vi "Window-Calibration toolbox_v9.vi"() -> ()   [LabVIEW 2020]
uses:
  Configuration code/Calibration/ToolBox/TypeDefs/Current Calibration Parameters.ctl
  Configuration code/Calibration/ToolBox/TypeDefs/ProcedureState.ctl
  Typedefs/Objective selector control enum.ctl
  <vilib>/vision/Image Controls.llb/IMAQ Image.ctl
  Configuration code/Calibration/ToolBox/TypeDefs/Incre-decr button.ctl
  Configuration code/Calibration/ToolBox/TypeDefs/Procedure_State.ctl
  Configuration code/Calibration/ToolBox/TypeDefs/Control Plane.ctl
  <vilib>/vision/Management.llb/Cast Image 2 Method.ctl
  Typedefs/HW config states enum.ctl
  Configuration code/Calibration/ToolBox/TypeDefs/data and image buffer fgv actions.ctl
  Typedefs/Shutter Function Enum.ctl
  Peripherals Control/XYZ Stage/Typedefs/XYZ stage data.ctl
  Peripherals Control/XYZ Stage/Typedefs/XYZ stage states.ctl
  Peripherals Control/XYZ Stage/Typedefs/XYZ channel ring.ctl
  Typedefs/Top level VI states.ctl
  Global Variables/General Globals.vi
  Configuration code/Calibration/Globals/gl_Calibration globals.vi
  Global Variables/gl_UI Ctrl Refs.vi
  <resource>/objmgr/IMAQImage.rc
  <vilib>/GPower/Array/GPArray.lvlib
  Global Variables/gl_Queues.vi
  <vilib>/vision/NI_Vision_Development_Module.lvlib
  <vilib>/GPower/Array/Library/Create/Random/CreateRandomI8.vi
panel:
  in  "Operation":T1(ring)
  in  "Exit":bool
  in  "Z Norm":bool
  in  "Signal Channel":enum16{"Red", "Green"}(ring)
  in  "Current Objective":T2="Olympus  20X"
  in  "Tab 2":T3(tab) caption="Calibration Tab"
  in  "Tab Control":T4(tab)
  in  "Freeze Core Image":bool
  out "Core Image":T5(plugin-control)
  in  "Core image":cluster{"Numeric":dbl, "Numeric":dbl}(slide)={"Numeric"=0.0, "Numeric"=1810.4210526315792} scale=0.0..4095.0
  in  "CH2":bool caption="CH"
  in  "Filter Type":T6(ring)
  out "Mean Value":sgl format="%.2f"
  in  "Mov. Avg":bool
  out "Histogram":T7(graph)
  out "Core Image frozen":T5(plugin-control)
  in  "Frozen core image intensity":cluster{"Numeric":dbl, "Numeric":dbl}(slide)={"Numeric"=0.0, "Numeric"=1810.4210526315792} scale=0.0..4095.0
  out "Core Image Filtered":T5(plugin-control)
  in  "Core image filtered":cluster{"Numeric":dbl, "Numeric":dbl}(slide)={"Numeric"=0.0, "Numeric"=1810.4210526315792} scale=0.0..255.0
  in  "AOL Controls Tab":T8(tab)
  in  "FOV":sgl(slide)=100.0 min=10 max=500 step=1 scale=25.0..500.0
  in  "Frame size":u16(slide)=256 min=2 max=2048 step=1 scale=2.0..2048.0
  in  "Dwell Time":dbl(slide)=0.1 min=0.05 max=0.4 step=0.05 scale=0.05..0.4
  in  "X Centre":sgl(slide) scale=-1.0..1.0 scale format="%#_2f"
  in  "Y Centre":sgl(slide) caption="Y centre" scale=-1.0..1.0 scale format="%#_2f"
  in  "AOLZ":sgl(slide) scale=-300.0..300.0 scale format="%#_2f"
  in  "Sum X":T9 step=0.1
  in  "Sum Y":T9 step=0.1
  in  "Sums Incr":dbl=0.1 caption="+/-" step=0.1
  in  "Diff X":T9 step=0.1
  in  "Diff Y":T9 step=0.1
  in  "Diffs Incr":dbl=0.1 caption="+/-"
  in  "Distortion Corr.":T9 step=0.1
  in  "DC Incr":dbl=0.1 caption="+/-"
  in  "X Angle":dbl(knob) min=0.0 max=359.9 step=0.1
  in  "Y Angle":dbl(knob)
  in  "Z Angle":dbl(knob)
  in  "Current Calibration Parameters":T10 {"Slip Cycle" step=0.1; "Samples to Wait after Trigger" step=0.1; "X_norm to um_scaling" step=0.1; "Z_norm to um_scaling" step=0.1; "Distortion Correction" step=0.1; "Diff Y" step=0.1; "Diff X" step=0.1; "Sum Y" step=0.1; "Sum X" step=0.1}
  in  "Incr":dbl=0.1 caption="+/-"
  in  "Plot":bool
  in  "Sort":bool
  in  "By":enum16{"Z", "X", "Y"}(ring)
  in  "Core Intensity 2":T11(tab) caption="Calibration Tab"
  out "Intensity":i16[][](graph)
  in  "Intensity Graph colour palette":cluster{dbl, "Color Box":u32}[](array[cluster])=[{1000.0, "Color Box"=16714752}, {750.0, "Color Box"=15859456}, {500.0, "Color Box"=65289}, {250.0, "Color Box"=983260}, {0.0, "Color Box"=14418124}]
  in  "core Intensity Graph colour palette":cluster{dbl, "Color Box":u32}[](array[cluster])=[{1000.0, "Color Box"=16714752}, {750.0, "Color Box"=15859456}, {500.0, "Color Box"=65289}, {250.0, "Color Box"=983260}, {0.0, "Color Box"=14418124}]
  out "Core Intensity":i16[][](graph)
  in  "Add images to buffer":bool
  in  "Saved Pos":i32[](listbox)
  in  "Add reference":bool
  in  "Clear all":bool
  in  "Clear selected":bool
  in  "Save to file":bool
  in  "Measure":bool
  in  "Tab Control 2":enum32{"Page 1", "Page 2"}(tab)
  out "Frozen image":T5(plugin-control)
  in  "Frozen Image intensity":cluster{i16, i16}(slide)={0, 2048} scale=0.0..4095.0
  in  "Image Buffer 1":i32(listbox)
  in  "Snap save":bool
  in  "Sweep":enum16{"Dwell Time", "SWAT"}(ring)
  out "Y Scaling":cluster{"X":dbl, "Y":dbl}[](graph)
  out "X Scaling":cluster{"X":dbl, "Y":dbl}[](graph)
  out "Z Scaling":cluster{"X":dbl, "Y":dbl}[](graph)
  in  "Reload":bool
  in  "Save config.ini":bool
  out "X":sgl format="X:%#_g"
  out "Y":sgl format="Y:%#_g"
  out "Z":sgl format="Z:%#_g"
  out "Procedure":T12
  out "Z plane exec time":u32
  out "error out 7":errorcluster
  out "error out 6":errorcluster
  out "Circles Data":T13(array[cluster])
  out "error out 8":errorcluster
  out "error out 5":errorcluster
  out "error out 3":errorcluster
  out "error out 4":errorcluster
  out "error out 2":errorcluster
  out "error out 10":errorcluster
  in  "Calibrate":bool
  in  "Test":bool
  in  "Sequence":bool
  in  "miniStep size":dbl=100.0 format="%#_g µm"
  out "UL":dbl=100.0 format="%#_g µm"
  out "LL":dbl=100.0 format="%#_g µm"
  out "mini steps":dbl=100.0
  out "New Image":T5
  in  "Freeze and plot":bool
  in  "sample dtype":dbl
  out "Stage Zeroed ?":bool
  out "Motor Z values":i32[](array[numeric])
  out "AOL Z values":i32[](array[numeric])
  out "Stage Zeroed ? 2":bool
  in  "Freeze Image":bool
  out "LB data full":string[][](array[string])
  out "LB data":string[][](array[string])
  out "Nb Circles":i32
  out "error out 9":errorcluster
  out "Intensity Graph":i16[][](graph)
  out "Image Pixels (I16)":i16[][](array[numeric])
  out "Progress":u8(slide) scale=0.0..21.0
  out "error out":errorcluster
  in  "Auto Focus":bool
  in  "Message_FrontPanel":string
  in  "Cancel":bool
  in  "Abort":bool
  in  "Next":bool
  in  "N":i32=512
  out "Stop_Ind":bool
  in  "Calibration Tab":T14(tab)
  in  "CH1":bool caption="CH"
  in  "Overlay\ncore":bool
  in  "Live Image intensity":cluster{i16, i16}(slide)={0, 2048} scale=0.0..4095.0
  in  "Visible(Grid)":bool
  in  "Grid Lines":u32=2 min=2 max=10 step=1
  out "Image":T5(plugin-control)
  out "Focal Plane":sgl format="Z:%#_g"
  in  "Set focal plane":bool
  in  "Natural Plane":bool
  in  "Move Up":bool
  in  "Move Down":bool
  in  "Z Step Size":dbl=100.0 format="%#_g µm"
  out "Stage XYZ Position":cluster{"X":sgl, "Y":sgl, "Z":sgl}
  in  "Zero Stage":bool
  out "X Res.":i32
  out "Y Res.":i32
  in  "Up":bool
  in  "Left":bool
  in  "Right":bool
  in  "Down":bool
  in  "Return":bool
  in  "XY Step Size":dbl=100.0 format="%#_g µm"
  in  "Core extraction size":i32 caption="Core size"
  in  "X offset":i32
  in  "Y offset":i32
  out "Array":T5[](array[plugin-control])
  out "Analysis Graph":cluster{"X":dbl, "Y":dbl}[](graph)
  out "PSF Plot":cluster{"X":dbl, "Y":dbl}[](graph)
  out "PSF Image":T5(plugin-control)
  in  "Objectives":string(tree)
  out "String":string
  out "Calibration.ini Path":path
  out "Calibration.ini":string
  in  "Step details":string
  in  "Step No":T15(ring)
  in  "Pockels Cell Value for pointing mode":dbl
  in  "auto-set pockel":bool
  in  "Calibration_min":dbl
  in  "Calibration_max":dbl
  in  "Search_min":dbl
  in  "Search_max":dbl
  in  "Testing Range (Norm)_max":dbl=1.0
  in  "Testing Range (Norm)_min":dbl=-1.0
  in  "Auto Calibration":bool
  in  "Measure PSF":bool
  in  "Calibration test type":T16(ring)
  in  "Calibration type":T17(ring)
  # "PROTOTYPE ONLY"
  # "This utility is under development, please report any \nissues to the contact details provided on github"
  # "12"
  # "0"
  # "2"
  # "8"
  # "0"
  # "2"
  # "PLACEHOLDER"
  # "Note :  Files will be saved in C:\\Support Files\\Calibration Data directory\nin pos_data_{date}_{time}.csv format"
  # "Current XYZ Stage Position"
  # "Natural Focal Plane Z motor position must\n be set to Zero before starting."
  # "Calibration Options"
  # "Maximal Search Range"
  # "to"
  # "(for sums &\ndiffs only)"
  # "Calibration Range from"
  # "to"
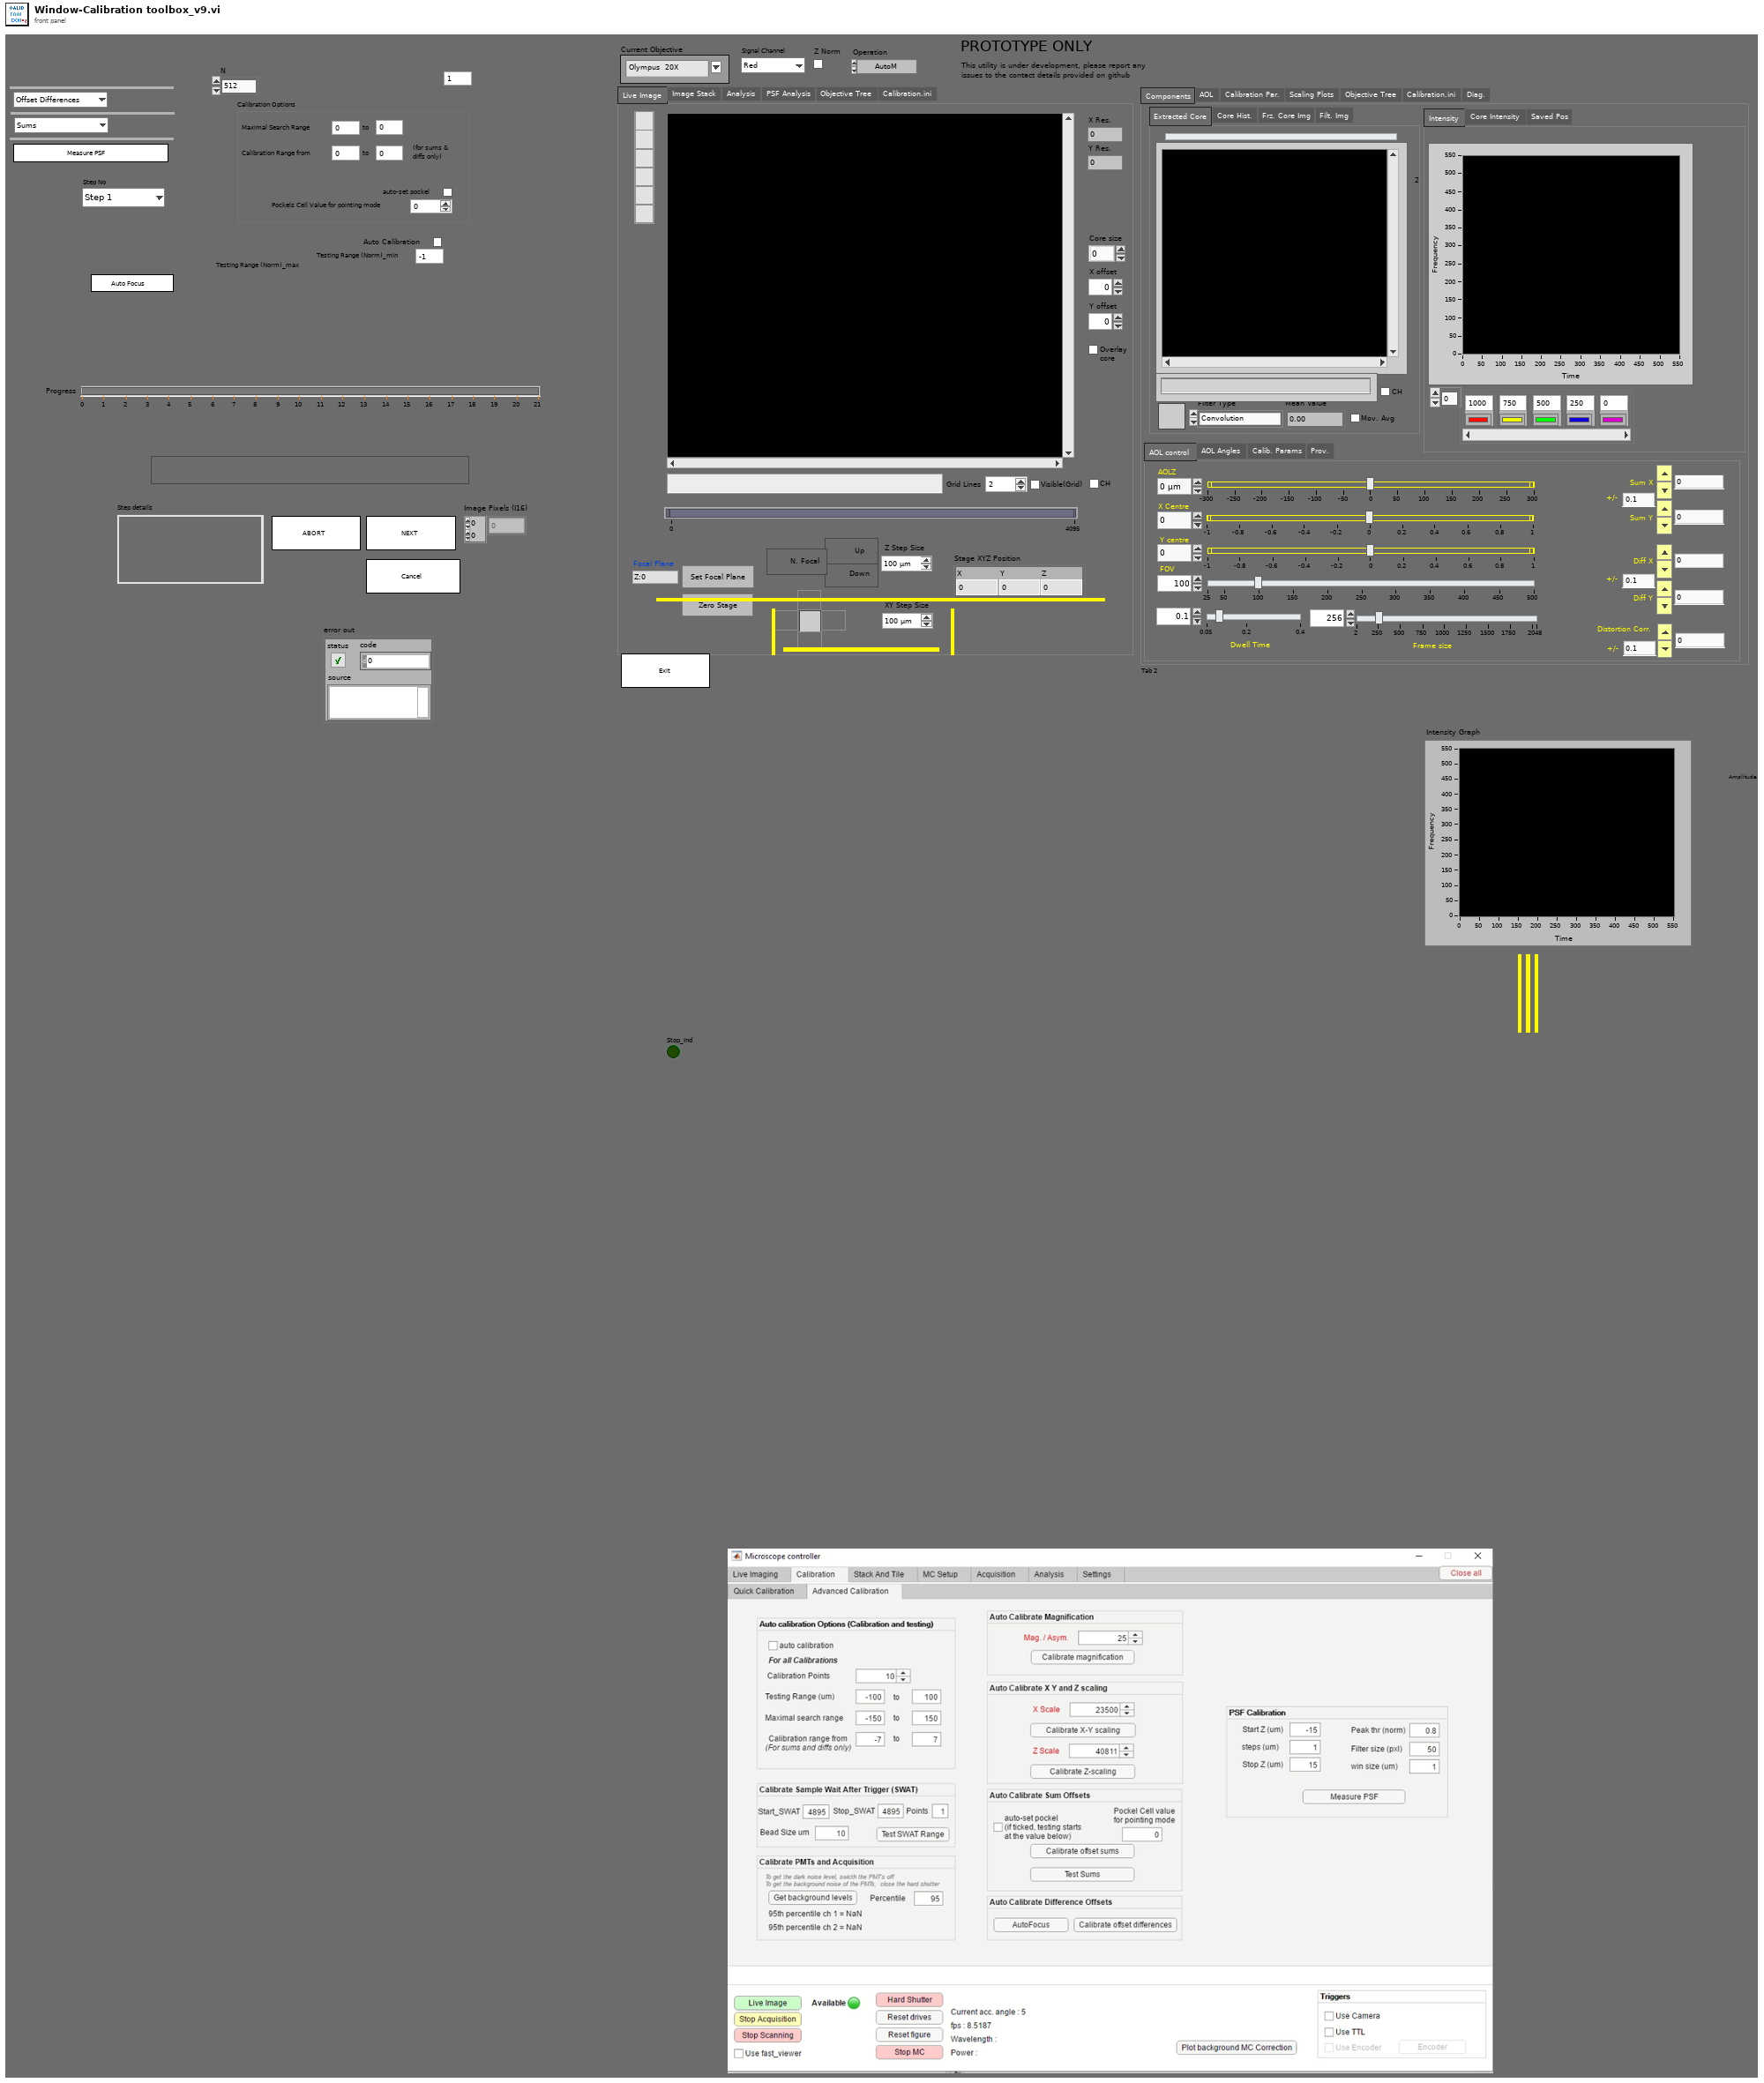
[diagram p1: front panel]
types:
  T1 = enum32{"AutoM", "Close", "Dilate", "Erode", "Gradient", "Gradient out", "Gradient in", "Hit miss", "Open", "PClose", "POpen", "Thick", "Thin"}
  T2 = typedef "Objective selector control enum.ctl" = string
  T3 = enum32{"Components", "AOL", "Calibration Par.", "Scaling Plots", "Objective Tree", "Calibration.ini", "Diag."}
  T4 = enum32{"Extracted Core", "Core Hist.", "Frz. Core Img", "Filt. Img"}
  T5 = typedef "IMAQ Image.ctl" = refnum<image>
  T6 = enum16{"Convolution", "Differentiation", "Gradient", "Prewitt", "Roberts", "Sigma", "Sobel"}
  T7 = cluster{"Starting Value":sgl, "Incremental Value":sgl, "Histogram":u32[]}
  T8 = enum32{"AOL control", "AOL Angles", "Calib. Params", "Prov."}
  T9 = typedef "Incre-decr button.ctl" = dbl
  T10 = typedef "Current Calibration Parameters.ctl" = cluster{"Sum X":dbl, "Sum Y":dbl, "Diff X":dbl, "Diff Y":dbl, "Distortion Correction":dbl, "Z_norm to um_scaling":dbl, "X_norm to um_scaling":dbl, "Samples to Wait after Trigger":dbl, "Slip Cycle":dbl}
  T11 = enum32{"Intensity", "Core Intensity ", "Saved Pos"}
  T12 = typedef "ProcedureState.ctl" = enum16{"Measure", "Calibrate", "Sequence", "Test"}
  T13 = cluster{"Pos. X":i32, "Pos. Y":i32, "Radius":i32, "Core Area":i32}[]
  T14 = enum32{"Live Image", "Image Stack", "Analysis", "PSF Analysis", "Objective Tree", "Calibration.ini"}
  T15 = enum16{"Step 1", "Step 2", "Step 3", "Step 4", "Step 5", "Step 6", "Step 7", "Step 8", "Step 9"}
  T16 = enum16{"Sums", "Diffs and Distortion", "Dwell Times"}
  T17 = enum16{"Offset Differences", "Magnification", "Offset Sums", "X-Y Scaling", "Z-Scaling"}
  T18 = typedef "Image Type" = u32
  T19 = enum32{"Invalid", "Standard", "Closed", "Hidden", "Minimized", "Maximized"}
  T20 = typedef "data and image buffer fgv actions.ctl" = enum16{"Initialise", "Add Image to buffer", "Read Image buffer", "Edit specific data", "Delete selected image", "Clear all images"}
  T21 = typedef "HW config states enum.ctl" = enum16{"Load from file", "Save to file", "Save backup", "Write all", "Read all", "Write XY stage settings", "Write DAQ FPGA settings", "Write Control FPGA settings", "Write Phys Channels", "Write System Config", "Write HW Config", "Save System Config", "Save HW Config", "Clear", "Compare from file"}
  T22 = enum8{"Enabled", "Disabled", "Disabled and Grayed Out"}
  T23 = enum16{"Initialise", "Load from file", "Save to file", "Read", "Write"}
  T24 = typedef "Shutter Function Enum.ctl" = enum16{"Open Shutter", "Close Shutter"}
  T25 = enum32{"Bad", "Idle", "Run top level", "Running"}
  T26 = typedef "Live graph data queue ref.ctl" = refnum<queue>
  T27 = enum32{"Image", "Image Stack", "Analysis", "PSF Analysis", "Objective Tree", "Calibration.ini"}
  T28 = typedef "Calibration config.ctl" = cluster{"Current Objective":string, "Objective Settings":T29[], "PreChirper Values Preset ?":bool, "PreChirper Settings":T30[], "PreChirper Constants":T31}
  T29 = typedef "Objective Config.ctl" = cluster{"Name":string, "Sum X":dbl, "Sum Y":dbl, "Diff X":dbl, "Diff Y":dbl, "Distortion Correction":dbl, "Z_norm to um_scaling":dbl, "X_norm to um_scaling":dbl, "Calibrated Wavelength":dbl}
  T30 = typedef "Prechirper Cal Config.ctl" = cluster{"Wavelength":i32, "Prism 1":i32, "Prism 2":i32}
  T31 = typedef "PreChirper constants.ctl" = cluster{"a 1":i32, "b 1":i32, "c 1":i32, "a 2":i32, "b 2":i32, "c 2":i32, "lmin":i32, "lmax":i32}
  T32 = typedef "System Configuration.ctl" = cluster{"Laser wavelength (nm)":dbl, "DAQ FPGA System":T33, "Control system":T34}
  T33 = typedef "DAQ FPGA system config.ctl" = cluster{"Clock Freq (MHz) ":dbl, "Samples Wait after Trigger":u16, "AOD fill":u16, "StartupDelay":i32, "Slip Cycle (clock cycles)":u32, "Add Cycle":bool}
  T34 = typedef "CTRL system config.ctl" = cluster{"AOD 1 Amplitude":i16, "AOD 2 Amplitude":i16, "AOD 3 Amplitude":i16, "AOD 4 Amplitude":i16, "AOD 5 Amplitude":i16, "AOD 6 Amplitude":i16, "T0 (ns)":dbl, "Ta (ns)":dbl, "Data Time Interval (ns)":dbl, "Ctrl FPGA Clock (MHz)":dbl}
  T35 = typedef "UI ctrl refs cluster.ctl" = cluster{"Top level VI path":path, "Top level VI ref":refnum<vi>, "User menu ref":refnum<k9>, "Sub Panel control":refnum<vi>, "Imaging Param Tab":refnum<vi>, "Occurrence-Start drivers":refnum<k4>, "Occurrence-Speed logging initialised":refnum<k4>, "Occurrence-XYZ stage initialised":refnum<k4>, "Exit button":refnum<vi>, "Status ind":refnum<vi>, "Set as origin":refnum<vi>, "Speed Logging":refnum<vi>, "Time Lapse":refnum<vi>, "Live Imaging":refnum<vi>, "AOL Z Stack":refnum<vi>, "Motor Z Stack":refnum<vi>, "Funct Acq button":refnum<vi>, "Hard Shutter":refnum<vi>, "Virtual Shutter":refnum<vi>, "Laser Power":refnum<vi>, "AOL Mode":refnum<vi>, "Frame Size":refnum<vi>, "Field of View":refnum<vi>, "Dwell Time":refnum<vi>, "Zoom":refnum<vi>, "AOL Z":refnum<vi>, "Objective":refnum<vi>, "Axis":refnum<vi>, "Paths & Names":refnum<vi>, "Experiment folder path (ind.)":refnum<vi>, "Last State (Ind.)":refnum<vi>, "Averages":refnum<vi>, "Angle (degrees)":refnum<vi>, "X centre":refnum<vi>, "Y centre":refnum<vi>, "Plane Mode":refnum<vi>, "# Planes":refnum<vi>, "Z Start":refnum<vi>, "Z Stop":refnum<vi>, "Z Step":refnum<vi>, "PMT 1":refnum<vi>, "PMT 2":refnum<vi>, "Stage XYZ Position":refnum<vi>, "Pockels@Z Start":refnum<vi>, "Pockels@Z Stop":refnum<vi>, "Obtain Z Start":refnum<vi>, "Obtain Z Stop":refnum<vi>, "Live stim.trig.period":refnum<vi>, "Live stim.trig.enable":refnum<vi>, "Movement Correction":refnum<vi>, "Load Reference Image":refnum<vi>, "XY Stage Move":refnum<vi>, "MovCor Cluster":refnum<vi>, "RefDAQParam":refnum<vi>, "Funct. Acq. Pockels Modulation":refnum<vi>, "Ref Laser Power":refnum<vi>, "Enable Video Recording":refnum<vi>, "Video Record-Live Imaging":refnum<vi>, "Video Record-Funct acq":refnum<vi>, "Reference Source":refnum<vi>, "AOL Z-stack Chirps Ready (ind)":refnum<vi>, "Target time between mov.cor. ref triggers (ms)":refnum<vi>, "Funct. Acq. Ref frame save":refnum<vi>, "Tracking button":refnum<vi>, "Show ref plots window":refnum<vi>, "Center freq ind (nm)":refnum<vi>, "Pickup mode (ind)":refnum<vi>, "Logging queue (ind)":refnum<vi>, "Back aperture power (ind.)":refnum<vi>, "Power after objective (ind.)":refnum<vi>, "Switch user":refnum<vi>, "Ls1 Conn. Status":refnum<vi>, "Ls1Tuning Status":refnum<vi>, "Ls1 Faults":refnum<vi>, "Ls1 Connection":refnum<vi>, "Ls1 Mode":refnum<vi>, "Ls1 POWER [mW]":refnum<vi>, "Ls1Shutter":refnum<vi>, "Ls1 Wavelength":refnum<vi>, "Ls1 Note":refnum<vi>, "Ls1 Confirm Wav":refnum<vi>, "Ls1 PreChrp Prism1":refnum<vi>, "Ls1 PreChrp Prism2":refnum<vi>, "Ls1 wav top Ind":refnum<vi>, "Ls1 power top Ind":refnum<vi>, "Ls1 Pump peak Hold":refnum<vi>, "Ls1 Status Ind":refnum<vi>, "Ls1 wav cancel":refnum<vi>, "Experiment Type":refnum<vi>, "Biology Information":refnum<vi>, "Camera recording status":refnum<vi>, "Optimise Obj. Pos.":refnum<vi>}
  T36 = typedef "AOL Z cal process refs.ctl" = cluster{"This VI":refnum<vi>, "Abort (ind)":refnum<vi>, "Next (ind)":refnum<vi>, "Cancel":refnum<vi>, "Next":refnum<vi>, "Message":refnum<vi>, "Progress":refnum<vi>}
  T37 = typedef "Frame Size.ctl" = u16
  T38 = typedef "Control Plane.ctl" = enum16{"XY-X", "XY-Y", "Z"}
  T39 = typedef "Procedure_State.ctl" = cluster{"Procedure":T12, "Parameter":T38, "Symmetric":bool}
  T40 = typedef "XYZ stage states.ctl" = enum16{"Dequeue", "Initialize", "Read Position", "Read Speed Setting", "Move", "Set Max Speed", "Reset Axis", "Stop all movement"}
  T41 = typedef "XYZ channel ring.ctl" = string
  T42 = typedef "XYZ stage data.ctl" = cluster{"Command":T40, "Channel":T41, "X":sgl, "Y":sgl, "Z":sgl, "Speed":i32, "Zero":bool, "Use acknowledgement?":bool}
  T43 = typedef "Top level VI states.ctl" = enum16{"None", "Initialise UI", "<STACK PROTOCOL STATES>", "AOL Zstack-START", "AOL Zstack-STOP", "Motor Zstack-START", "Motor Zstack-STOP", "Parameter Sweep-START", "Parameter Sweep-STOP", "<ACQUISITION PROTOCOL STATES> ", "Functional Acquisition-START", "Functional Acquisition-STOP", "Single Plane Acquisition-START", "Single Plane Acquisition-STOP", "Volume Acquisition-START", "Volume Acquisition-STOP", "<LIVE IMAGING PROTOCOL STATES>", "Live Imaging-START", "Live Imaging-STOP", "Live Plane Imaging-START", "Live Plane Imaging-STOP", "Live Volume Imaging-START", "Live Volume Imaging-STOP", "<MOVEMENT CORRECTION PROTOCOL STATES>", "EXIT"}
  T44 = enum16{"open", "replace", "create", "open or create", "replace or create", "replace or create with confirmation"}
  T45 = typedef "AOL_Globals.ctl" = cluster{"Imaging Protocol":T46, "Number of POI":u16, "Number of Miniscans":u16, "Number of Trials":u16, "Number of Cycles ":u64, "# Averaged Frames":u16, "Laser power (%)":u8, "Pockels (V)":dbl, "Acquisition Length (sec)":dbl, "Fill time (us)":dbl, "POI Dwell time (us)":dbl, "Miniscan Dwell time per pixel (us)":dbl, "PMT 1":dbl, "PMT 2":dbl, "Back Apperture (mA)":dbl, "Frame Size":T37, "Center Frequency":dbl, "Field of View (um)":dbl, "Field of View (norm)":dbl, "DwellTime (us)":dbl, "Ref Dwell Time (us)":dbl, "Wavelength (nm)":dbl, "Zoom":dbl, "AOL Z":dbl, "AOL Mode":T47, "GridXY":dbl, "GridZ":dbl, "TriggerPeriod (sec)":dbl, "Number of Pixels in Miniscan":u16, "Experiment folder path":path, "X centre":dbl, "Y centre":dbl, "Angle (degrees)":dbl, "Angle Xs (degrees)":dbl, "Angle Ys (degrees)":dbl, "Plane Mode":T48, "Threshold":u16[], "Regenerate Chirps":bool, "Rectangle ROI length (pixels)":u16, "Rectangle ROI height (pixels)":u16, "AOD fill":u16, "StartupDelay":i32, "Samples Wait after Trigger":u16, "Slip Cycle":u32, "Add Cycle":bool, "Functional Mode":T49, "Z Start":dbl, "Z Stop":dbl, "# Planes":i32, "Total Pixels":i32, "Variable Miniscan Pixels":u16[], "Use Variable Length":bool, "Use Variable Resolution":bool, "Laser power (%) at Z Start":u8, "Laser power (%) at Z Stop":u8, "Ref Z Step":i8}
  T46 = typedef "Imaging Protocols enum.ctl" = enum16{"AOL Z-Stack", "Motor Z Stack", "Parameter Sweep", "Functional Acquisition", "Single Plane Acquisition", "Volume Acquisition", "Live Imaging", "Live Plane Imaging", "Live Volume Imaging"}
  T47 = typedef "AOL modes.ctl" = enum16{"Raster", "Structural", "Pointing", "Mini Scan", "Alignment"}
  T48 = typedef "Plane Mode.ctl" = u16
  T49 = typedef "Functional Mode.ctl" = enum16{"Point", "Line", "Patch", "Plane", "Volume"}
  T50 = typedef "Live imaging queue element.ctl" = cluster{"Red channel":T5, "Green channel":T5, "Ref Red channel":T5, "Ref Green channel":T5, "Mov cor":bool}
  T51 = typedef "IMAQ Circle" = cluster{"Center X":i32, "Center Y":i32, "Inner Radius":i32, "Outer Radius":i32, "Start Angle":dbl, "End Angle":dbl}
  T52 = enum32{"Differentiation", "Gradient", "Prewitt", "Roberts", "Sigma", "Sobel"}
  T53 = typedef "Cast Image 2 Method.ctl" = u32
  T54 = typedef "ROI Descriptor" = cluster{"Global Rectangle":i32[], "Contours":cluster{"ID":enum32{"External", "Internal"}, "Type":u32, "Coordinates":i32[]}[]}
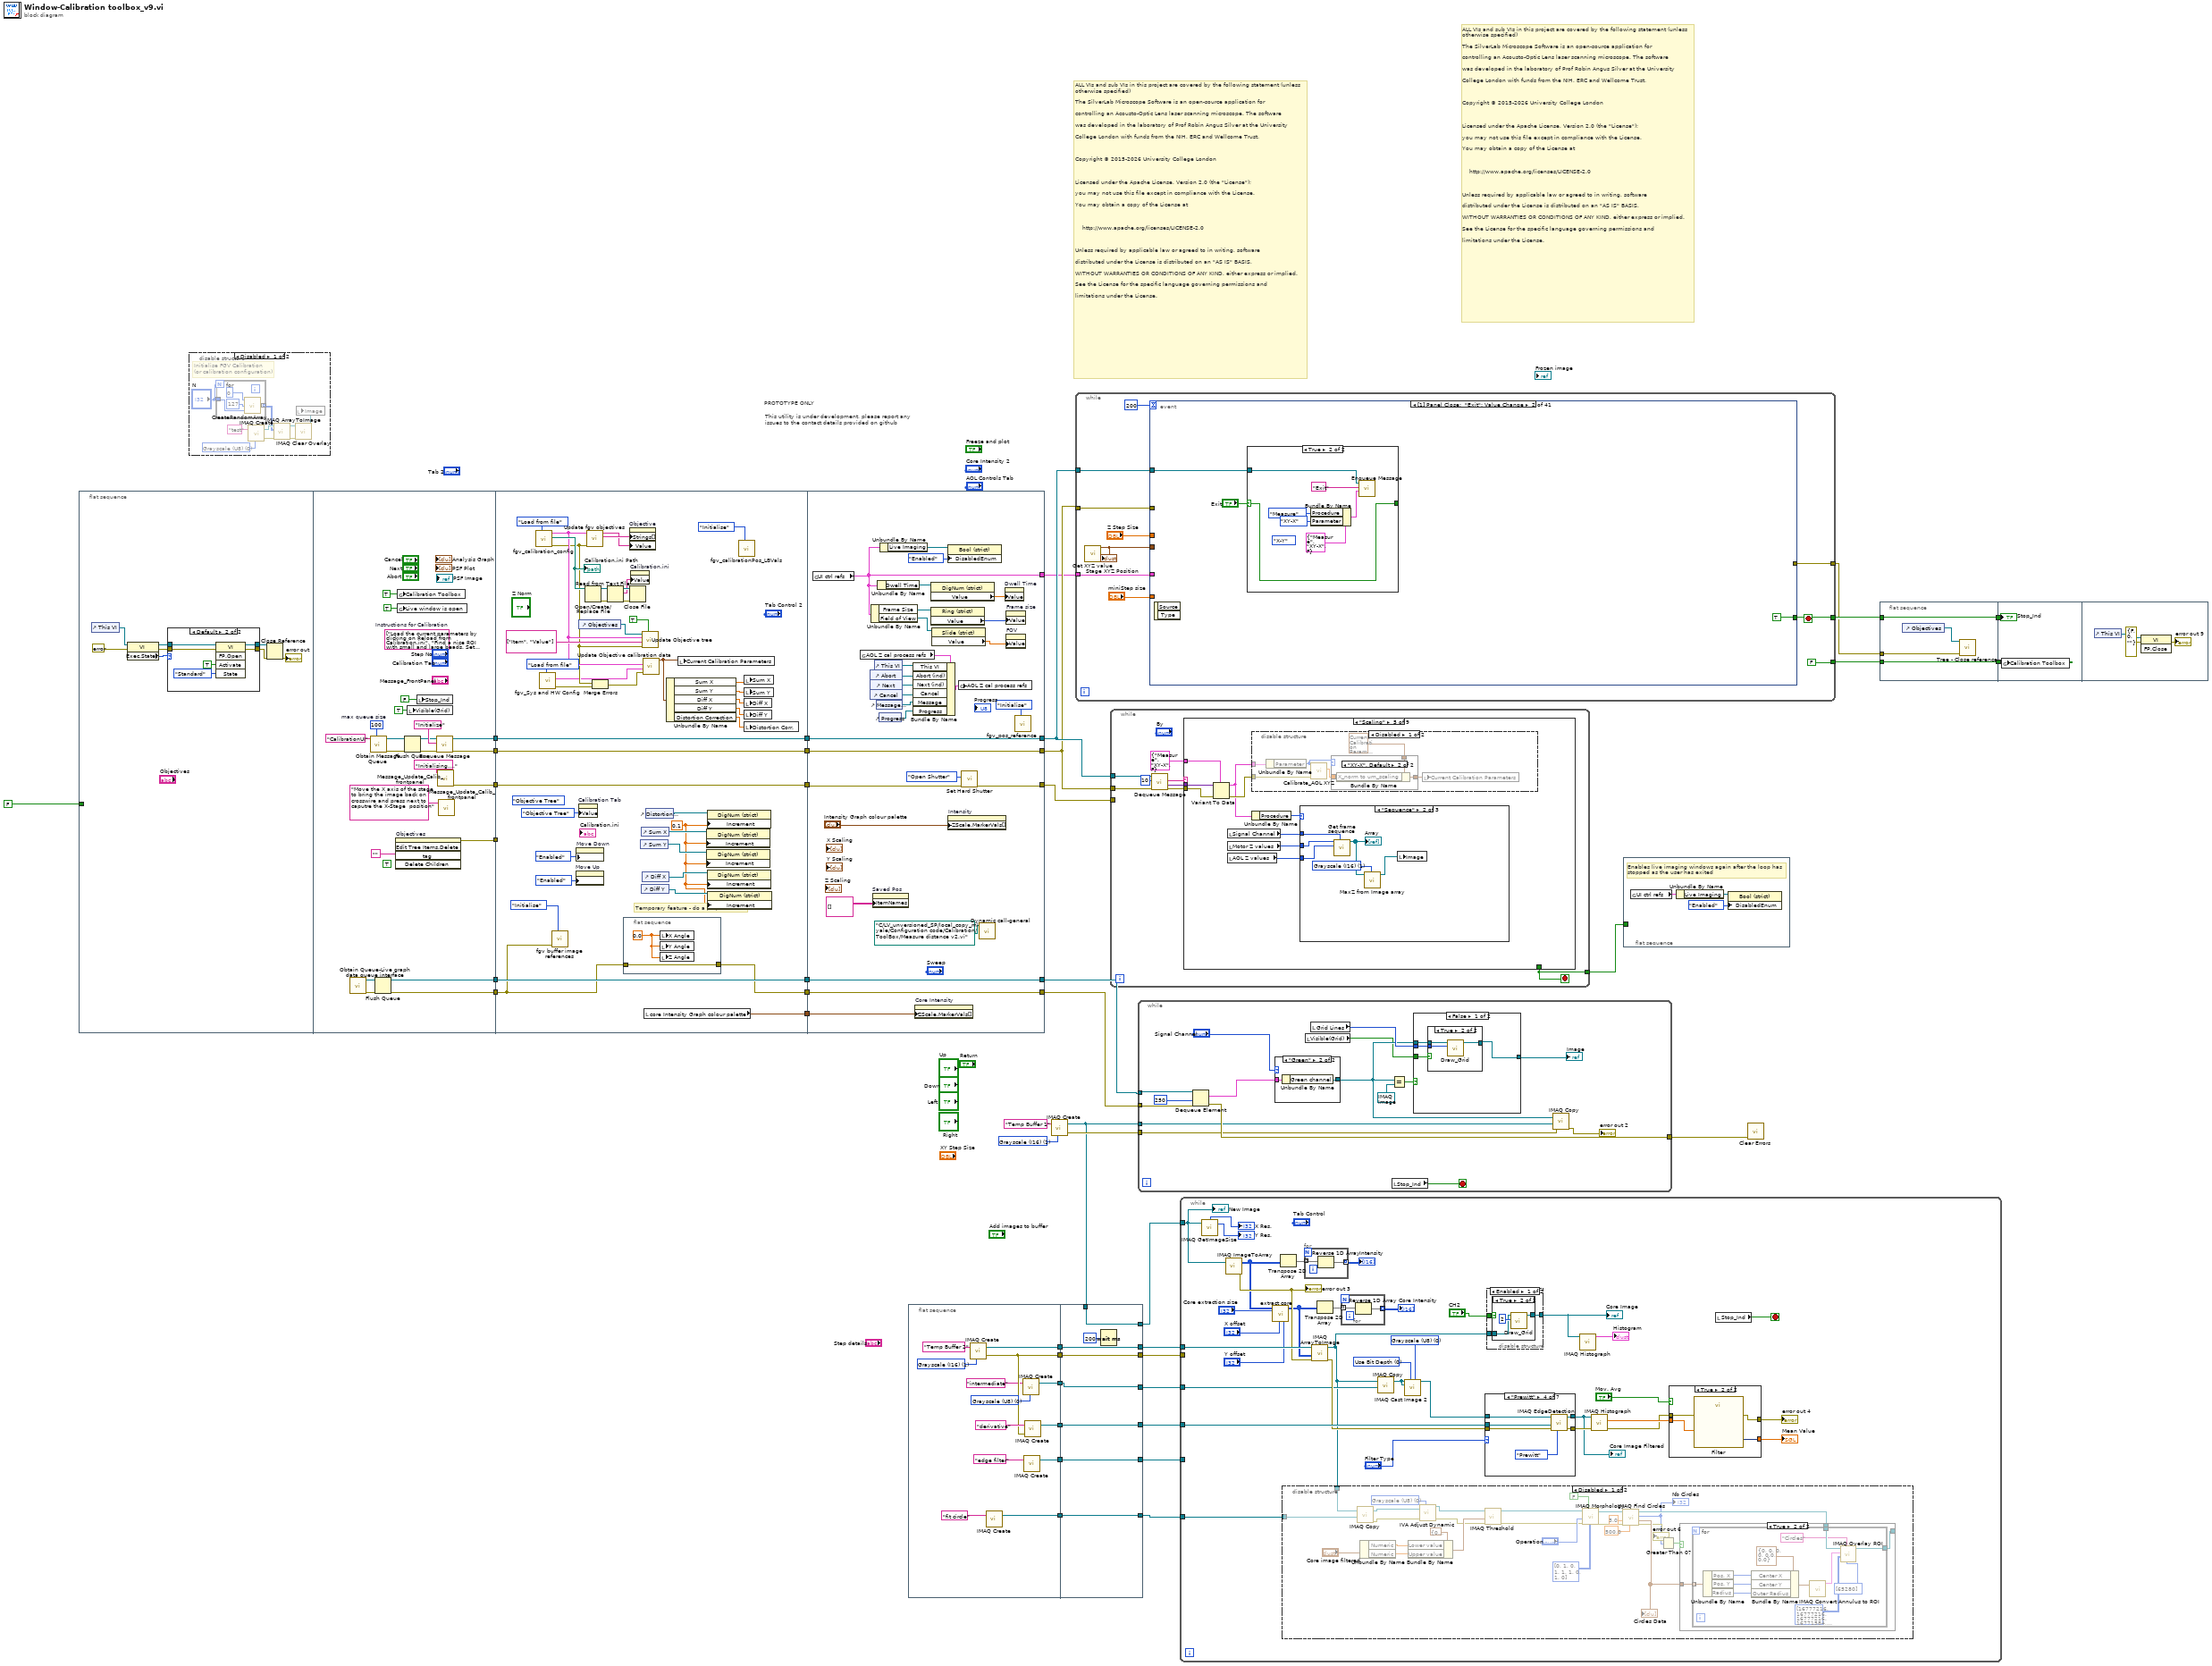
[diagram p0: block diagram]
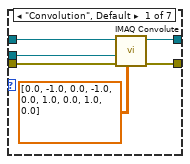
[diagram p7: hidden frame]
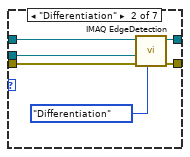
[diagram p8: hidden frame]
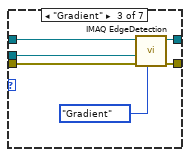
[diagram p9: hidden frame]
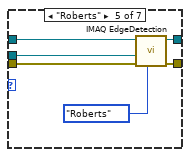
[diagram p10: hidden frame]
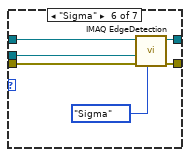
[diagram p11: hidden frame]
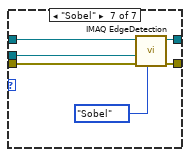
[diagram p12: hidden frame]
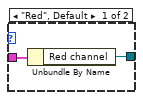
[diagram p14: hidden frame]
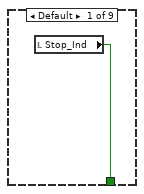
[diagram p18: hidden frame]
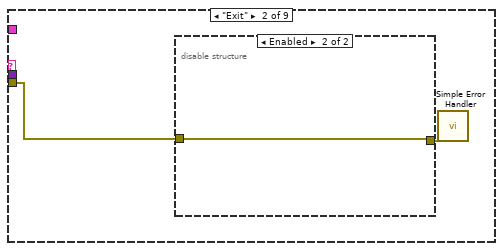
[diagram p19: hidden frame]
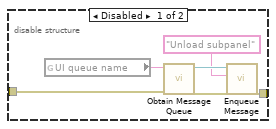
[diagram p20: hidden frame]
diagram:
  w23 = T18 1 items=["Grayscale (U8)", "Grayscale (I16)", "Grayscale (SGL)", "Complex (CSG)", "RGB (U32)", "HSL (U32)", "RGB (U64)", "Grayscale (U16)"] ("Image Type")
  # "ALL VIs and sub VIs in this project are covered by the following statement (unless \notherwise specified)\n\nThe SilverLab Microscope Software is an open-source application for\n\ncontrolling an Acousto-Optic Lens laser scanning microscope. The software\n\nwas developed in the laboratory of Prof Robin Angus Silver at the University\n\nCollege London with funds from the NIH, ERC and Wellcome Trust.\n\n \n\nCopyright © 2015-2026 University College London\n\n \n\nLicensed under the Apache License, Version 2.0 (the \"License\");\n\nyou may not use this file except in compliance with the License.\n\nYou may obtain a copy of the License at\n\n \n\n    http://www.apache.org/licenses/LICENSE-2.0\n\n \n\nUnless required by applicable law or agreed to in writing, software\n\ndistributed under the License is distributed on an \"AS IS\" BASIS,\n\nWITHOUT WARRANTIES OR CONDITIONS OF ANY KIND, either express or implied.\n\nSee the License for the specific language governing permissions and\n\nlimitations under the License."
  # "This utility is under development, please report any \nissues to the contact details provided on github"
  # "PROTOTYPE ONLY"
  # "ALL VIs and sub VIs in this project are covered by the following statement (unless \notherwise specified)\n\nThe SilverLab Microscope Software is an open-source application for\n\ncontrolling an Acousto-Optic Lens laser scanning microscope. The software\n\nwas developed in the laboratory of Prof Robin Angus Silver at the University\n\nCollege London with funds from the NIH, ERC and Wellcome Trust.\n\n \n\nCopyright © 2015-2026 University College London\n\n \n\nLicensed under the Apache License, Version 2.0 (the \"License\");\n\nyou may not use this file except in compliance with the License.\n\nYou may obtain a copy of the License at\n\n \n\n    http://www.apache.org/licenses/LICENSE-2.0\n\n \n\nUnless required by applicable law or agreed to in writing, software\n\ndistributed under the License is distributed on an \"AS IS\" BASIS,\n\nWITHOUT WARRANTIES OR CONDITIONS OF ANY KIND, either express or implied.\n\nSee the License for the specific language governing permissions and\n\nlimitations under the License."
  n1 = flat-sequence {
    tunnel: FALSE -> [_]
    tunnel: [w74] -> w37
    tunnel: [w73] -> w35
    tunnel: [w71] -> w33
    tunnel: [w64] -> w31
    tunnel: [w62] -> w29
    tunnel: [w61] -> w25
    tunnel: w37 -> [w123]
    tunnel: [w123] -> w36
    tunnel: w35 -> [w122]
    tunnel: [w122] -> w34
    tunnel: w33 -> [w121]
    tunnel: [w121] -> w32
    tunnel: w31 -> [w120]
    tunnel: [w120] -> w30
    tunnel: w29 -> [w84]
    tunnel: [w91] -> w28
    tunnel: w25 -> [_]
    tunnel: [w98] -> w19
    tunnel: [w151] -> w17
    tunnel: [w152] -> w18
    tunnel: [w132] -> w39
    tunnel: [w153] -> w41
    tunnel: [w154] -> w42
    tunnel: w36 -> [w154]
    tunnel: w34 -> [w153]
    tunnel: w32 -> [w133]
    tunnel: w30 -> [w152]
    tunnel: w28 -> [w151]
    tunnel: [w131] -> w27
    tunnel: w19 -> [w139]
    frame #0 {
      n2 = control-ref of="This VI"() -> (w48:refnum<vi>)
      n3 = property class="VI"(reference=w48, error in=errorcluster {"status"=FALSE, "code"=0, "source"=""} ("error in (no error)")) -> (reference out=w47:refnum<vi>, error out=w46:errorcluster, "Exec.State"=w44:T25)
      n4 = case shown="Default" w44 {
        tunnel: [w53 w54] -> w51
        tunnel: [w52 w59] -> w50
        tunnel: w47 -> [w53 w56]
        tunnel: w46 -> [w52 w55]
        frame "Run top level" {
        }
        frame Default {
          n5 = invoke class="VI" method="FP.Open"(reference=w56, error in=w55, "Activate"=TRUE ("Activate?"), "State"=T19."Standard") -> (reference out=w54:refnum<vi>, error out=w59:errorcluster)  [unwired: 1 in, 3 out]
        }
      }
      n6 = Close Reference(reference=w51, error in (no error)=w50) -> (error out=→"error out":errorcluster)
    }
    frame #1 {
      (unwired) TRUE ("Delete Children?")
      w76 = 100  # max queue size
      (unwired) string[] ["Load the current parameters by clicking on Reload from Calibration.ini", "Find a nice ROI with small and large beads. Set PMT at 500 and adjust pockels", "Test FOV gives a sharp, single peak with Auto Focus. If yes, zero the stage. Otherwise change ROI", "Use 'Test Diffs and distortion' AND ' Test Sum' to see if the rig needs calibration for differences or sums.", "Process to teh necessary calibrations. If the performances are suboptimal, change ROI or incease laser", "If the results are bad, you can restore the previous settings by clicking on Reload from calibration.ini", "If calibration fails repetitively, try another magnification, laser pwer or FOV size.", "If calibration crashes in mid-process, go to Acquisition tab, reset drives and set the stage back to [0,0,0]. If you were in pointing mode, set teh mode toggie back to raster. Then check the pockels values."]  # Instructions for Calibration
      n7 = call "Obtain Queue-Live graph data queue interface.vi"() -> ("error out"=w65:errorcluster, "Live graphs queue"=w66:T26)  [unwired: 10 in]
      n8 = call "Obtain Message Queue.vi"("max queue size (-1, unlimited)"=w76, "Queue name"="CalibrationUI") -> ("error out"=w78:errorcluster, "Message Queue"=w80:refnum<queue>)  [unwired: 8 in]
      n9 = Flush Queue(queue=w66, error in (no error)=w65) -> (queue out=w64:T26, error out=w62:errorcluster)  [unwired: 1 out]
      n10 = invoke on="Objectives" class="Tree (strict)" method="Edit Tree Items.Delete"("tag"="") -> (error out=w61:errorcluster)  [unwired: 4 in, 4 out]
      n11 = global write "General Globals.vi" "Calibration Toolbox"(TRUE ("Calibration Toolbox")) -> ()
      n12 = global write "General Globals.vi" "Live window is open"(TRUE ("Live window is open")) -> ()
      n13 = Flush Queue(queue=w80, error in (no error)=w78) -> (queue out=w79:refnum<queue>, error out=w77:errorcluster)  [unwired: 1 out]
      n14 = local write "Visible(Grid)"(TRUE ("Visible(Grid)")) -> ()
      n15 = local write "Stop_Ind"(FALSE ("Stop_Ind")) -> ()
      n16 = call "Enqueue Message.vi"("error in (no error)"=w77, "Message"="Initialize", "Queue"=w79) -> ("error out"=w73:errorcluster, "Queue out"=w74:refnum<queue>)  [unwired: 7 in]
      n17 = call "Message_Update_Calib_frontpanel.vi"("Message"="Initialising....") -> ("error out"=w71:errorcluster)  [unwired: 10 in]
      n18 = call "Message_Update_Calib_frontpanel.vi"("Message"="Move the X axis of the stage to bring the image back on crosswire and press next to caputre the X-Stage  position") -> ()  [unwired: 10 in, 1 out]
    }
    frame #2 {
      w85 = 0.1 ("Data Entry Limits:Increment")
      (unwired) T27."Objective Tree" ("Calibration Tab")
      # "Temporary feature - do a proper initialise"
      n19 = call "fgv_calibration_config.vi"("Cal config ops"=T23."Load from file") -> ("error out"=w103:errorcluster, "Config file path"=w108:path, "Config cluster OUT"=w107:T28)  [unwired: 8 in]
      "Calibration.ini Path" <- w108
      n20 = call "fgv_Sys and HW Config.vi"("Function"=HW_config_states_enum."Load from file") -> ("error out"=w102:errorcluster, "System Config OUT"=w100:T32)  [unwired: 8 in, 1 out]
      n21 = call "fgv buffer image references.vi"("Actions"=data_and_image_buffer_fgv_actions."Initialise", "error in (no error)"=w84) -> ()  [unwired: 7 in, 7 out]
      n22 = property on="Move Up" class="Bool"("DisabledEnum"=T22."Enabled" ("Disabled")) -> ()  [unwired: 2 in, 2 out]
      n23 = property on="Move Down" class="Bool"("DisabledEnum"=T22."Enabled" ("Disabled")) -> ()  [unwired: 2 in, 2 out]
      n24 = property on="Calibration Tab" class="TabCtl (strict)"("Value"=T14."Objective Tree" ("Calibration Tab")) -> ()  [unwired: 2 in, 2 out]
      n25 = control-ref of="Objectives"() -> (w111:refnum<vi>)
      n26 = Open/Create/Replace File(file path (use dialog)=w108) -> (refnum out=w116:refnum<file>, error out=w115:errorcluster)  [unwired: 5 in, 1 out]
      n27 = call "Update fgv objectives.vi"("error in (no error)"=w103, "Config cluster IN"=w107) -> ("Available Objectives"=w113:string[], "Current Objective"=w112:string)  [unwired: 7 in, 1 out]
      n28 = Merge Errors(w103, w102) -> (w101:errorcluster)
      n29 = Read from Text File(file (use dialog)=w116, error in=w115) -> (refnum out=w117:refnum<file>, text=w114:string, error out=w118:errorcluster)  [unwired: 2 in, 1 out]
      n30 = flat-sequence {
        tunnel: [w124] -> w91
        tunnel: w84 -> [w124]
        frame #0 {
          w125 = 0.0
          n31 = local write "X Angle"(w125) -> ()
          n32 = local write "Y Angle"(w125) -> ()
          n33 = local write "Z Angle"(w125) -> ()
        }
      }
      n34 = property on="Objective" class="CmbBox (strict)"("Strings[]"=w113, "Value"=w112) -> ()  [unwired: 2 in, 2 out]
      n35 = Close File(refnum=w117, error in=w118) -> ()  [unwired: 2 out]
      n36 = property on="Calibration.ini" class="Str"("Value"=w114) -> ()  [unwired: 2 in, 2 out]
      n37 = control-ref of="Sum Y"() -> (w86:refnum<vi>)
      n38 = control-ref of="Sum X"() -> (w87:refnum<vi>)
      n39 = control-ref of="Diff Y"() -> (w88:refnum<vi>)
      n40 = call "Update Objective tree.vi"("Visible Items:Column Headers Visible"=TRUE, "error in (no error)"=w103, "Column Header Strings[]"=string[] ["Item", "Value"], "Config cluster IN"=w107, "TreeControl in"=w111) -> ()  [unwired: 6 in, 1 out]
      n41 = control-ref of="Diff X"() -> (w89:refnum<vi>)
      n42 = call "Update Objective calibration data.vi"("error in (no error)"=w101, "System Config"=w100, "Config cluster OUT"=w107) -> ("Current Calibration Parameters out"=w97:T10)  [unwired: 7 in, 1 out]
      n43 = local read "core Intensity Graph colour palette"() -> (w98:cluster{dbl, "Color Box":u32}[])
      n44 = control-ref of="Distortion Corr."() -> (w90:refnum<vi>)
      n45 = Unbundle By Name(w97) -> ("Sum X"=w96:dbl, "Sum Y"=w95:dbl, "Diff X"=w94:dbl, "Diff Y"=w93:dbl, "Distortion Correction"=w92:dbl)
      n46 = local write "Current Calibration Parameters"(w97) -> ()
      n47 = property class="DigNum (strict)"(reference=w87, "Increment"=w85) -> ()  [unwired: 1 in, 2 out]
      n48 = property class="DigNum (strict)"(reference=w86, "Increment"=w85) -> ()  [unwired: 1 in, 2 out]
      n49 = property class="DigNum (strict)"(reference=w90, "Increment"=w85) -> ()  [unwired: 1 in, 2 out]
      n50 = property class="DigNum (strict)"(reference=w89, "Increment"=w85) -> ()  [unwired: 1 in, 2 out]
      n51 = property class="DigNum (strict)"(reference=w88, "Increment"=w85) -> ()  [unwired: 1 in, 2 out]
      n52 = call "fgv_calibrationPos_LBVals.vi"("ACtions"=enum16{"Initialise", "Get", "Set"}."Initialise") -> ()  [unwired: 9 in, 2 out]
      n53 = local write "Sum X"(w96) -> ()
      n54 = local write "Sum Y"(w95) -> ()
      n55 = local write "Diff X"(w94) -> ()
      n56 = local write "Diff Y"(w93) -> ()
      n57 = local write "Distortion Corr."(w92) -> ()
    }
    frame #3 {
      n58 = global read "gl_UI Ctrl Refs.vi" "UI ctrl refs"() -> (w131:T35)
      n59 = global read "gl_Calibration globals.vi" "AOL Z cal process refs"() -> (w145:T36)
      n60 = control-ref of="Abort"() -> (w144:refnum<vi>)
      n61 = control-ref of="Next"() -> (w150:refnum<vi>)
      n62 = control-ref of="Cancel"() -> (w146:refnum<vi>)
      n63 = Unbundle By Name(w131) -> ("Frame Size"=w130:refnum<vi>, "Field of View"=w128:refnum<vi>)
      n64 = property on="Saved Pos" class="MCListbox (strict)"("ItemNames"=string[][] []) -> ()  [unwired: 2 in, 2 out]
      n65 = control-ref of="This VI"() -> (w149:refnum<vi>)
      n66 = control-ref of="Message_FrontPanel"() -> (w147:refnum<vi>)
      n67 = Unbundle By Name(w131) -> ("Dwell Time"=w136:refnum<vi>)
      n68 = control-ref of="Progress"() -> (w141:refnum<vi>)
      n69 = Unbundle By Name(w131) -> ("Live Imaging"=w143:refnum<vi>)
      n70 = Bundle By Name(cluster=w145, "This VI"=w149, "Abort (ind)"=w144, "Next (ind)"=w150, "Cancel"=w146, "Message"=w147, "Progress"=w141) -> (w148:T36)
      n71 = property on="Core Intensity" class="IntGraph (strict)"("ZScale.MarkerVals[]"=w139) -> ()  [unwired: 2 in, 2 out]
      n72 = property class="DigNum (strict)"(reference=w136) -> ("Value"=w135:dbl)  [unwired: 1 in, 2 out]
      n73 = property class="Ring (strict)"(reference=w130) -> ("Value"=w129:T37)  [unwired: 1 in, 2 out]
      n74 = property class="Slide (strict)"(reference=w128) -> ("Value"=w127:sgl)  [unwired: 1 in, 2 out]
      n75 = property class="Bool (strict)"(reference=w143, "DisabledEnum"=T22."Enabled" ("Disabled")) -> ()  [unwired: 1 in, 2 out]
      n76 = property on="Intensity" class="IntGraph (strict)"("ZScale.MarkerVals[]"="Intensity Graph colour palette") -> ()  [unwired: 2 in, 2 out]
      n77 = global write "gl_Calibration globals.vi" "AOL Z cal process refs"(w148) -> ()
      n78 = call "Set Hard Shutter.vi"("Error In"=w133, "Shutter Function"=Shutter_Function_Enum."Open Shutter") -> ("Error Out"=w132:errorcluster)  [unwired: 9 in]
      n79 = call "Dynamic call-general.vi"("vi path"=path "C:/LV_unversioned_SP/local_copy_ml_yale/Configuration code/Calibration/ToolBox/Measure distance v2.vi") -> ()  [unwired: 10 in, 1 out]
      n80 = property on="Dwell Time" class="Slide (strict)"("Value"=w135) -> ()  [unwired: 2 in, 2 out]
      n81 = property on="Frame size" class="Slide (strict)"("Value"=w129) -> ()  [unwired: 2 in, 2 out]
      n82 = property on="FOV" class="Slide (strict)"("Value"=w127) -> ()  [unwired: 2 in, 2 out]
      n83 = call "fgv_pos_reference.vi"("State"=enum16{"Initialise", "Write", "Read", "Clear"}."Initialise") -> ()  [unwired: 8 in, 3 out]
    }
  }
  n84 = disable-structure shown="Disabled" {
    frame Disabled {
      w162 = T18 0 items=["Grayscale (U8)", "Grayscale (I16)", "Grayscale (SGL)", "Complex (CSG)", "RGB (U32)", "HSL (U32)", "RGB (U64)", "Grayscale (U16)"] ("Image Type")
      # "Initialise FGV Calibration\n(or calibration configuration)"
      n85 = for {
        N: "N" -> [_]
        tunnel: [w165] -> w159 mode=indexing
        tunnel: "N" -> [w164]
        n86 = call-poly <vilib>:"CreateRandomArray.vi"("N"=w164, "Maximum value"=i8 127, "Minimum value"=i8 0) -> ("Created array"=w165:i8[])
      }
      n87 = call "IMAQ Create"("Image Name"="test", "Image Type"=w162) -> ("New Image"=w160:T5, "error out"=w161:errorcluster)  [unwired: 3 in]
      n88 = call "IMAQ ArrayToImage"("error in (no error)"=w161, "Image Pixels (U8)"=w159, "Image"=w160) -> ("error out"=w156:errorcluster, "Image Out"=w157:T5)  [unwired: 7 in]
      n89 = call "IMAQ Clear Overlay"("error in (no error)"=w156, "Image"=w157) -> ("Image Out"=w155:T5)  [unwired: 8 in, 1 out]
      n90 = local write "Image"(w155) -> ()
    }
    frame Enabled {
    }
  }
  n91 = flat-sequence {
    tunnel: [w178] -> w16
    tunnel: [w176] -> w15
    tunnel: [w175] -> w12
    tunnel: [w172] -> w10
    tunnel: [w170] -> w8
    tunnel: [w168] -> w6
    tunnel: [w187] -> w20
    tunnel: [w188] -> w21
    tunnel: w16 -> [w188]
    tunnel: w15 -> [w187]
    tunnel: [w185] -> w14
    tunnel: w13 -> [w185]
    tunnel: [w184] -> w11
    tunnel: w12 -> [w184]
    tunnel: [w183] -> w9
    tunnel: w10 -> [w183]
    tunnel: w8 -> [w182]
    tunnel: [w182] -> w7
    tunnel: w6 -> [w181]
    tunnel: [w181] -> w5
    frame #0 {
      w173 = T18 0 items=["Grayscale (U8)", "Grayscale (I16)", "Grayscale (SGL)", "Complex (CSG)", "RGB (U32)", "HSL (U32)", "RGB (U64)", "Grayscale (U16)"] ("Image Type")
      w180 = T18 1 items=["Grayscale (U8)", "Grayscale (I16)", "Grayscale (SGL)", "Complex (CSG)", "RGB (U32)", "HSL (U32)", "RGB (U64)", "Grayscale (U16)"] ("Image Type")
      n92 = call "IMAQ Create"("Image Name"="Temp Buffer 2", "Image Type"=w180) -> ("New Image"=w178:T5, "error out"=w176:errorcluster)  [unwired: 3 in]
      n93 = call "IMAQ Create"("Image Name"="fit circle") -> ("New Image"=w168:T5)  [unwired: 4 in, 1 out]
      n94 = call "IMAQ Create"("Image Name"="intermediate", "Image Type"=w173) -> ("New Image"=w172:T5)  [unwired: 3 in, 1 out]
      n95 = call "IMAQ Create"("Image Name"="edge filter") -> ("New Image"=w170:T5)  [unwired: 4 in, 1 out]
      n96 = call "IMAQ Create"("Image Name"="derivative", "error in (no error)"=w176) -> ("New Image"=w175:T5)  [unwired: 3 in, 1 out]
    }
    frame #1 {
      n97 = Wait (ms)(milliseconds to wait=u32 200) -> ()  [unwired: 1 out]
    }
  }
  n98 = call "IMAQ Create"("Image Name"="Temp Buffer 1", "Image Type"=w23) -> ("New Image"=w13:T5, "error out"=w22:errorcluster)  [unwired: 3 in]
  n99 = while {
    tunnel: [w198] -> w43
    tunnel: w42 -> [w197]
    tunnel: w41 -> [w194]
    tunnel: [FALSE ("Calibration Toolbox")] -> w40
    tunnel: w27 -> [w193]
    tunnel: [w192] -> w1
    stop <- w198 stop-if-true
    n100 = call "Get XYZ value.vi"() -> ("Stage XYZ Position"=w189:cluster{"X":sgl, "Y":sgl, "Z":sgl})  [unwired: 11 in]
    "Stage XYZ Position" <- w189
    n101 = event shown="[1] Panel Close;  \"Exit\": Value Change" {
      selector: _ -> [_ _ _ _ _ _ _ _ _ _ _ _ _ _ _ _ _ _ _ _ _ _ _ _ _ _ _ _ _ _ _ _ _ _ _ _ _ _ _ _ _]
      dyn-events: _ -> [_ _ _ _ _ _ _ _ _ _ _ _ _ _ _ _ _ _ _ _ _ _ _ _ _ _ _ _ _ _ _ _ _ _ _ _ _ _ _ _ _]
      timeout: 200 -> [_ _ _ _ _ _ _ _ _ _ _ _ _ _ _ _ _ _ _ _ _ _ _ _ _ _ _ _ _ _ _ _ _ _ _ _ _ _ _ _ _]
      tunnel: [_ TRUE _ _ _ _ _ _ _ _ _ _ _ _ _ _ _ _ _ _ _ _ _ _ _ _ _ _ _ _ _ _ _ _ _ _ _ _ _ _ _] -> w198
      tunnel: w197 -> [_ w215 _ _ _ _ _ _ _ _ _ w467 w521 w573 _ w596 _ _ _ _ _ _ _ _ _ _ _ _ _ _ _ _ _ _ _ _ _ _ _ _ _]
      tunnel: w194 -> [_ _ _ _ _ _ _ _ _ _ _ _ _ _ _ _ _ _ _ _ _ _ _ _ w740 w763 _ _ _ _ _ _ _ _ _ _ _ _ _ _ _]
      tunnel: w193 -> [_ _ _ w243 _ w316 w359 w381 w405 w424 _ w465 w520 w563 _ _ _ _ _ _ _ _ _ _ _ _ _ _ _ _ _ _ _ _ _ _ _ _ _ _ _]
      tunnel: [_ _ _ _ _ w311 w356 w378 w402 w419 _ _ _ _ _ _ w602 _ _ _ _ _ _ _ w740 w761 _ _ _ _ _ _ _ _ _ _ _ _ _ _ _] -> w192
      tunnel: "Z Step Size" -> [w202 _ _ w231 w310 _ _ _ _ _ _ _ _ _ _ _ _ _ _ _ _ _ _ _ _ _ _ _ _ _ _ _ _ _ _ _ _ _ _ _ _]
      tunnel: "miniStep size" -> [w201 _ _ _ w306 _ _ _ _ _ _ _ _ _ _ _ _ _ _ _ _ _ _ _ _ _ _ _ _ _ _ _ _ _ _ _ _ _ _ _ _]
      tunnel: w189 -> [w200 _ w226 w230 _ _ _ _ _ _ _ _ _ _ _ _ _ _ _ _ _ _ _ _ w741 _ _ _ _ _ _ _ w808 _ _ _ _ _ _ _ _]
      event Timeout {
        n102 = event-data() -> ()  [unwired: 1 in, 3 out]
        n103 = First Call?() -> (First Call?: T/F=w203:bool)
        n104 = Unbundle By Name(w200) -> ("X"=→"X":sgl, "Y"=→"Y":sgl, "Z"=w199:sgl)
        "Z" <- w199
        n105 = case shown="False" w203 {
          tunnel: w202 -> [_ w213]
          tunnel: w201 -> [_ w212]
          tunnel: w199 -> [_ w206]
          frame False {
          }
          frame True {
            n106 = Absolute Value(x=w213) -> (abs(x)=w211:dbl)
            n107 = local write "Focal Plane"(w206) -> ()
            n108 = Negate(x=w211) -> (-x=w210:dbl)
            n109 = call "Calculate Z step size.vi"("Step"=w212, "Stop"=w210, "Start"=w211) -> ("AOL Z values"=w207:dbl[], "Motor Z values"=w208:i32[], "Number of steps"=w209:i32)  [unwired: 6 in]
            n110 = local write "LL"(w210) -> ()
            n111 = local write "UL"(w211) -> ()
            n112 = local write "AOL Z values"(w207) -> ()
            n113 = local write "mini steps"(w209) -> ()
            n114 = local write "Motor Z values"(w208) -> ()
          }
        }
      }
      event Panel Close; "Exit": Value Change {
        n115 = event-data() -> ()  [unwired: 1 in, 2 out]
        n116 = case shown="True" "Exit" {
          selector: "Exit" -> [w217 w218]
          tunnel: w215 -> [_ w224]
          tunnel: [w217 w218] -> _
          frame False {
          }
          frame True {
            (unwired) enum16{"X-Y", "Z"}."X-Y" ("Parameter")
            n117 = Bundle By Name(cluster=T39 {"Procedure"=enum."Measure", "Parameter"=enum."XY-X", "Symmetric"=FALSE} ("input cluster"), "Procedure"=ProcedureState."Measure", "Parameter"=Control_Plane."XY-X") -> (w221:T39)
            n118 = call "Enqueue Message.vi"("Message Data"=w221, "Message"="Exit", "Queue"=w224) -> ()  [unwired: 7 in, 2 out]
          }
        }
      }
      event "Set focal plane": Value Change {
        n119 = event-data() -> ()  [unwired: 1 in, 6 out]
        n120 = Unbundle By Name(w226) -> ("Z"=→"Focal Plane":sgl)
      }
      event "Move Up", "Move Down", "Natural Plane": Value Change {
        n121 = event-data() -> ("CtlRef"=w246:refnum<vi>)  [unwired: 1 in, 3 out]
        n122 = Unbundle By Name(w230) -> ("Z"=w229:sgl)
        n123 = Unbundle By Name(w243) -> ("AOL Z"=w242:refnum<vi>)
        n124 = property class="Bool"(reference=w246) -> (error out=w244:errorcluster, "Label.Text"=w245:string)  [unwired: 1 in, 1 out]
        n125 = flat-sequence {
          tunnel: w245 -> [w250]
          tunnel: w244 -> [w253]
          tunnel: [w252] -> w239
          tunnel: [w251] -> w237
          tunnel: [w250] -> w235
          tunnel: [w249] -> w232
          tunnel: w231 -> [w248]
          tunnel: w229 -> [w247]
          tunnel: w239 -> [w269]
          tunnel: [w269] -> w238
          tunnel: w237 -> [w268]
          tunnel: [w268] -> w236
          tunnel: w235 -> [w267]
          tunnel: [w267] -> w234
          tunnel: [w264] -> w233
          tunnel: w232 -> [w265]
          tunnel: [w263] -> w227
          tunnel: w238 -> [w278]
          tunnel: w236 -> [w277]
          tunnel: w242 -> [w276]
          tunnel: [w275] -> w241
          tunnel: w234 -> [w275]
          tunnel: w233 -> [w274]
          tunnel: [w274] -> w240
          tunnel: [w272] -> w228
          tunnel: w227 -> [w272]
          tunnel: w241 -> [w296]
          tunnel: w240 -> [w295]
          tunnel: w228 -> [w291]
          frame #0 {
            n126 = global read "gl_Calibration globals.vi" "AOL Z cal process refs"() -> (w249:T36)
            n127 = case shown="\"Natural Plane\", Default" w250 {
              tunnel: w253 -> [_ _ _]
              tunnel: w248 -> [_ w256 w261]
              tunnel: [0.0 ("Step Size") w259 w261] -> w251
              tunnel: [w254 w257 w260] -> w252
              tunnel: w247 -> [_ w258 w262]
              frame "Natural Plane", Default {
                n128 = local read "Focal Plane"() -> (w254:sgl)
              }
              frame "Move Up" {
                n129 = Add(x=w256, y=w258) -> (x+y=w257:dbl)
                n130 = Negate(x=w256) -> (-x=w259:dbl)
              }
              frame "Move Down" {
                n131 = Subtract(x=w262, y=w261) -> (x-y=w260:dbl)
              }
            }
          }
          frame #1 {
            n132 = Unbundle By Name(w265) -> ("Message"=w264:refnum<vi>)
            n133 = disable-structure shown="Disabled" {
              frame Disabled {
                w270 = T22."Disabled and Grayed Out" ("Disabled")
                n134 = property on="Move Up" class="Bool"("DisabledEnum"=w270) -> ()  [unwired: 2 in, 2 out]
                n135 = property on="Move Down" class="Bool"("DisabledEnum"=w270) -> ()  [unwired: 2 in, 2 out]
                n136 = property on="Natural Plane" class="Bool"("DisabledEnum"=w270) -> ()  [unwired: 2 in, 2 out]
              }
              frame Enabled {
              }
            }
            n137 = property class="Str"(reference=w264, "Value"="Adjusting...") -> ()  [unwired: 1 in, 2 out]
            n138 = Tick Count (ms)() -> (millisecond timer value=w263:u32)
          }
          frame #2 {
            n139 = disable-structure shown="Enabled" {
              disable-tunnel: [w288 errorcluster {"status"=FALSE, "code"=0, "source"=""} ("error in")] -> w282
              disable-tunnel: w277 -> [w287 _]
              disable-tunnel: w276 -> [w286 _]
              frame Disabled {
                n140 = property class="Slide (strict)"(reference=w286, "Value"=w287) -> (error out=w288:errorcluster)  [unwired: 1 in, 1 out]
                n141 = call "fgv_AOL_Globals Read.vi"() -> ("AOL_Globals"=w284:T45)  [unwired: 9 in, 2 out]
                n142 = Bundle By Name(cluster=w284, "AOL Z"=w287) -> (w285:T45)
                n143 = call "fgv_AOL_Globals Write.vi"("AOL_Globals"=w285) -> ()  [unwired: 10 in, 1 out]
              }
              frame Enabled {
              }
            }
            n144 = Bundle By Name(cluster=T42 {"Command"=enum."Initialize", "Channel"="Z", "X"=0.0, "Y"=0.0, "Z"=0.0, "Speed"=0, "Zero"=FALSE, "Use acknowledgement?"=TRUE} ("XYZ Stage data to queue"), "Command"=XYZ_stage_states."Move", "Channel"=T41 "Z", "Z"=w278, "Use acknowledgement?"=FALSE) -> (w283:T42)
            n145 = call "XYZ Stage-Command request module.vi"("error in"=w282, "Command"=XYZ_stage_states."Move", "XYZ Stage data to queue"=w283) -> ()  [unwired: 4 in, 5 out]
          }
          frame #3 {
            n146 = disable-structure shown="Disabled" {
              disable-tunnel: w296 -> [w297 _]
              frame Disabled {
                n147 = case shown="\"Natural Plane\", Default" w297 {
                  frame "Move Up" {
                    n148 = property on="Move Down" class="Bool"("DisabledEnum"=T22."Enabled" ("Disabled")) -> ()  [unwired: 2 in, 2 out]
                    n149 = property on="Move Up" class="Bool"("DisabledEnum"=T22."Disabled and Grayed Out" ("Disabled")) -> ()  [unwired: 2 in, 2 out]
                  }
                  frame "Move Down" {
                    n150 = property on="Move Up" class="Bool"("DisabledEnum"=T22."Enabled" ("Disabled")) -> ()  [unwired: 2 in, 2 out]
                    n151 = property on="Move Down" class="Bool"("DisabledEnum"=T22."Disabled and Grayed Out" ("Disabled")) -> ()  [unwired: 2 in, 2 out]
                  }
                  frame "Natural Plane", Default {
                    n152 = property on="Move Up" class="Bool"("DisabledEnum"=T22."Enabled" ("Disabled")) -> ()  [unwired: 2 in, 2 out]
                    n153 = property on="Move Down" class="Bool"("DisabledEnum"=T22."Enabled" ("Disabled")) -> ()  [unwired: 2 in, 2 out]
                  }
                }
              }
              frame Enabled {
              }
            }
            n154 = Tick Count (ms)() -> (millisecond timer value=w292:u32)
            n155 = Subtract(x=w292, y=w291) -> (x-y=→"Z plane exec time":u32)
            n156 = property on="Natural Plane" class="Bool"("DisabledEnum"=T22."Enabled" ("Disabled")) -> ()  [unwired: 2 in, 2 out]
            n157 = property class="Str"(reference=w295, "Value"="Done") -> ()  [unwired: 1 in, 2 out]
          }
        }
      }
      event "Z Step Size", "miniStep size": Value Change {
        n158 = event-data() -> ()  [unwired: 1 in, 6 out]
        n159 = Absolute Value(x=w310) -> (abs(x)=w309:dbl)
        "UL" <- w309
        n160 = Negate(x=w309) -> (-x=w308:dbl)
        "LL" <- w308
        n161 = call "Calculate Z step size.vi"("Step"=w306, "Stop"=w308, "Start"=w309) -> ("AOL Z values"=→"AOL Z values":dbl[], "Motor Z values"=→"Motor Z values":i32[], "Number of steps"=→"mini steps":i32)  [unwired: 6 in]
      }
      event "AOLZ", "X Centre", "Y Centre": Value Change {
        n162 = event-data() -> ("CtlRef"=w322:refnum<vi>, "NewVal"=w315:sgl)  [unwired: 1 in, 4 out]
        n163 = property class="Slide (strict)"(reference=w322) -> ("Label.Text"=w321:string)  [unwired: 1 in, 2 out]
        n164 = call "fgv_AOL_Globals Read.vi"() -> ("error out"=w317:errorcluster, "AOL_Globals"=w320:T45)  [unwired: 9 in, 1 out]
        n165 = case shown="\"X Centre\"" w321 {
          tunnel: w320 -> [w332 w337 w344 w350]
          tunnel: [w332 w335 w343 w348] -> w319
          tunnel: [w331 w336 w342 w349] -> w318
          tunnel: w317 -> [w331 w336 w342 w349]
          tunnel: w315 -> [_ w334 w339 w345]
          tunnel: w316 -> [_ w333 w341 w347]
          frame Default {
          }
          frame "AOLZ" {
            n166 = Unbundle By Name(w333) -> ("AOL Z"=w338:refnum<vi>)
            n167 = property class="Slide (strict)"(reference=w338, "Value"=w334) -> ()  [unwired: 1 in, 2 out]
            n168 = Bundle By Name(cluster=w337, "Y centre"=w334) -> (w335:T45)
          }
          frame "X Centre" {
            n169 = Unbundle By Name(w341) -> ("X centre"=w340:refnum<vi>)
            n170 = Bundle By Name(cluster=w344, "X centre"=w339) -> (w343:T45)
            n171 = property class="DigNum (strict)"(reference=w340, "Value"=w339) -> ()  [unwired: 1 in, 2 out]
          }
          frame "Y Centre" {
            n172 = Unbundle By Name(w347) -> ("Y centre"=w346:refnum<vi>)
            n173 = property class="DigNum (strict)"(reference=w346, "Value"=w345) -> ()  [unwired: 1 in, 2 out]
            n174 = Bundle By Name(cluster=w350, "Y centre"=w345) -> (w348:T45)
          }
        }
        n175 = call "fgv_AOL_Globals Write.vi"("error in (no error)"=w318, "AOL_Globals"=w319) -> ("error out"=w312:errorcluster)  [unwired: 9 in]
        n176 = flat-sequence {
          tunnel: w312 -> [w324]
          tunnel: [w323] -> w314
          tunnel: [w327] -> w313
          tunnel: w314 -> [w327]
          tunnel: w313 -> [w330]
          tunnel: [w329] -> w311
          frame #0 {
            n177 = call "Fire User Event - Next State.vi"("Error In"=w324, "\"UI Handler loop\" case to execute"=Top_level_VI_states."Live Imaging-STOP" ("event data / imaging mode")) -> ("Error Out"=w323:errorcluster)  [unwired: 9 in]
          }
          frame #1 {
            n178 = Wait (ms)(milliseconds to wait=u32 1000) -> ()  [unwired: 1 out]
          }
          frame #2 {
            n179 = call "Fire User Event - Next State.vi"("Error In"=w330, "\"UI Handler loop\" case to execute"=Top_level_VI_states."Live Imaging-START" ("event data / imaging mode")) -> ("Error Out"=w329:errorcluster)  [unwired: 9 in]
          }
        }
      }
      event "Dwell Time": Value Change {
        n180 = event-data() -> ("NewVal"=w351:dbl)  [unwired: 1 in, 5 out]
        n181 = Unbundle By Name(w359) -> ("Dwell Time"=w355:refnum<vi>)
        n182 = property class="DigNum (strict)"(reference=w355, "Value"=w351) -> (error out=w354:errorcluster)  [unwired: 1 in, 1 out]
        n183 = call "AOL Globals mode updater.vi"("error in"=w354) -> ("error out"=w353:errorcluster)  [unwired: 10 in]
        n184 = flat-sequence {
          tunnel: w353 -> [w362]
          tunnel: [w361] -> w352
          tunnel: w351 -> [w360]
          tunnel: [w365] -> w358
          tunnel: w352 -> [w366]
          tunnel: [w369] -> w357
          tunnel: w358 -> [w369]
          tunnel: w357 -> [w372]
          tunnel: [w371] -> w356
          frame #0 {
            n185 = call "fgv_AOL_Globals Read.vi"() -> ("AOL_Globals"=w364:T45)  [unwired: 9 in, 2 out]
            n186 = Bundle By Name(cluster=w364, "DwellTime (us)"=w360) -> (w363:T45)
            n187 = call "fgv_AOL_Globals Write.vi"("error in (no error)"=w362, "AOL_Globals"=w363) -> ("error out"=w361:errorcluster)  [unwired: 9 in]
          }
          frame #1 {
            n188 = call "Fire User Event - Next State.vi"("Error In"=w366, "\"UI Handler loop\" case to execute"=Top_level_VI_states."Live Imaging-STOP" ("event data / imaging mode")) -> ("Error Out"=w365:errorcluster)  [unwired: 9 in]
          }
          frame #2 {
            n189 = Wait (ms)(milliseconds to wait=u32 1000) -> ()  [unwired: 1 out]
          }
          frame #3 {
            n190 = call "Fire User Event - Next State.vi"("Error In"=w372, "\"UI Handler loop\" case to execute"=Top_level_VI_states."Live Imaging-START" ("event data / imaging mode")) -> ("Error Out"=w371:errorcluster)  [unwired: 9 in]
          }
        }
      }
      event "Frame size": Value Change {
        n191 = event-data() -> ("NewVal"=w376:u16)  [unwired: 1 in, 5 out]
        n192 = Unbundle By Name(w381) -> ("Frame Size"=w377:refnum<vi>)
        n193 = call "Manipulate frame size.vi"("Value"=w376, "Frame Size"=w377) -> ("error out"=w374:errorcluster, "Updated frame size"=w373:T37)  [unwired: 8 in]
        n194 = flat-sequence {
          tunnel: w374 -> [w383]
          tunnel: [w382] -> w375
          tunnel: w373 -> [w384]
          tunnel: [w387] -> w380
          tunnel: w375 -> [w388]
          tunnel: [w391] -> w379
          tunnel: w380 -> [w391]
          tunnel: w379 -> [w394]
          tunnel: [w393] -> w378
          frame #0 {
            n195 = call "fgv_AOL_Globals Read.vi"() -> ("AOL_Globals"=w386:T45)  [unwired: 9 in, 2 out]
            n196 = Bundle By Name(cluster=w386, "Frame Size"=w384) -> (w385:T45)
            n197 = call "fgv_AOL_Globals Write.vi"("error in (no error)"=w383, "AOL_Globals"=w385) -> ("error out"=w382:errorcluster)  [unwired: 9 in]
          }
          frame #1 {
            n198 = call "Fire User Event - Next State.vi"("Error In"=w388, "\"UI Handler loop\" case to execute"=Top_level_VI_states."Live Imaging-STOP" ("event data / imaging mode")) -> ("Error Out"=w387:errorcluster)  [unwired: 9 in]
          }
          frame #2 {
            n199 = Wait (ms)(milliseconds to wait=u32 1000) -> ()  [unwired: 1 out]
          }
          frame #3 {
            n200 = call "Fire User Event - Next State.vi"("Error In"=w394, "\"UI Handler loop\" case to execute"=Top_level_VI_states."Live Imaging-START" ("event data / imaging mode")) -> ("Error Out"=w393:errorcluster)  [unwired: 9 in]
          }
        }
      }
      event "FOV": Value Change {
        n201 = event-data() -> ("NewVal"=w397:sgl)  [unwired: 1 in, 5 out]
        n202 = Unbundle By Name(w405) -> ("Field of View"=w400:refnum<vi>, "Objective"=w399:refnum<vi>)
        n203 = property class="CmbBox"(reference=w399) -> ("Value"=w398:string)  [unwired: 1 in, 2 out]
        n204 = property class="Slide (strict)"(reference=w400, "Value"=w397) -> (error out=w396:errorcluster)  [unwired: 1 in, 1 out]
        n205 = call "Calculate acceptance angle.vi"("Objective"=w398, "FOV (true)"=w397) -> ("Acceptance Angle (mrad)"=w395:dbl)  [unwired: 8 in, 1 out]
        n206 = flat-sequence {
          tunnel: w396 -> [w408]
          tunnel: [w407] -> w401
          tunnel: w395 -> [w406]
          tunnel: [w411] -> w404
          tunnel: w401 -> [w412]
          tunnel: [w415] -> w403
          tunnel: w404 -> [w415]
          tunnel: w403 -> [w418]
          tunnel: [w417] -> w402
          frame #0 {
            n207 = call "fgv_AOL_Globals Read.vi"() -> ("AOL_Globals"=w410:T45)  [unwired: 9 in, 2 out]
            n208 = Bundle By Name(cluster=w410, "Field of View (norm)"=w406) -> (w409:T45)
            n209 = call "fgv_AOL_Globals Write.vi"("error in (no error)"=w408, "AOL_Globals"=w409) -> ("error out"=w407:errorcluster)  [unwired: 9 in]
          }
          frame #1 {
            n210 = call "Fire User Event - Next State.vi"("Error In"=w412, "\"UI Handler loop\" case to execute"=Top_level_VI_states."Live Imaging-STOP" ("event data / imaging mode")) -> ("Error Out"=w411:errorcluster)  [unwired: 9 in]
          }
          frame #2 {
            n211 = Wait (ms)(milliseconds to wait=u32 1000) -> ()  [unwired: 1 out]
          }
          frame #3 {
            n212 = call "Fire User Event - Next State.vi"("Error In"=w418, "\"UI Handler loop\" case to execute"=Top_level_VI_states."Live Imaging-START" ("event data / imaging mode")) -> ("Error Out"=w417:errorcluster)  [unwired: 9 in]
          }
        }
      }
      event "X Angle", "Y Angle", "Z Angle": Value Change {
        n213 = event-data() -> ("CtlRef"=w430:refnum<vi>, "NewVal"=w423:dbl)  [unwired: 1 in, 4 out]
        n214 = property class="Knob (strict)"(reference=w430) -> ("Label.Text"=w429:string)  [unwired: 1 in, 2 out]
        n215 = call "fgv_AOL_Globals Read.vi"() -> ("error out"=w428:errorcluster, "AOL_Globals"=w425:T45)  [unwired: 9 in, 1 out]
        n216 = case shown="\"Z Angle\"" w429 {
          tunnel: [w440 w441 w447 w452] -> w427
          tunnel: w428 -> [w440 w441 w447 w452]
          tunnel: [w439 w442 w446 w453] -> w426
          tunnel: w425 -> [w439 w444 w448 w454]
          tunnel: w424 -> [_ _ _ w450]
          tunnel: w423 -> [_ w443 w445 w449]
          frame Default {
          }
          frame "X Angle" {
            n217 = Bundle By Name(cluster=w444, "Angle Xs (degrees)"=w443) -> (w442:T45)
          }
          frame "Y Angle" {
            n218 = Bundle By Name(cluster=w448, "Angle Ys (degrees)"=w445) -> (w446:T45)
          }
          frame "Z Angle" {
            n219 = Unbundle By Name(w450) -> ("Angle (degrees)"=w451:refnum<vi>)
            n220 = property class="DigNum (strict)"(reference=w451, "Value"=w449) -> ()  [unwired: 1 in, 2 out]
            n221 = Bundle By Name(cluster=w454, "Angle (degrees)"=w449) -> (w453:T45)
          }
        }
        n222 = call "fgv_AOL_Globals Write.vi"("error in (no error)"=w427, "AOL_Globals"=w426) -> ("error out"=w422:errorcluster)  [unwired: 9 in]
        n223 = flat-sequence {
          tunnel: w422 -> [w432]
          tunnel: [w431] -> w420
          tunnel: [w435] -> w421
          tunnel: w420 -> [w435]
          tunnel: w421 -> [w438]
          tunnel: [w437] -> w419
          frame #0 {
            n224 = call "Fire User Event - Next State.vi"("Error In"=w432, "\"UI Handler loop\" case to execute"=Top_level_VI_states."Live Imaging-STOP" ("event data / imaging mode")) -> ("Error Out"=w431:errorcluster)  [unwired: 9 in]
          }
          frame #1 {
            n225 = Wait (ms)(milliseconds to wait=u32 100) -> ()  [unwired: 1 out]
          }
          frame #2 {
            n226 = call "Fire User Event - Next State.vi"("Error In"=w438, "\"UI Handler loop\" case to execute"=Top_level_VI_states."Live Imaging-START" ("event data / imaging mode")) -> ("Error Out"=w437:errorcluster)  [unwired: 9 in]
          }
        }
      }
      event "Save config.ini": Value Change {
        n227 = event-data() -> ()  [unwired: 1 in, 6 out]
      }
      event "Calibrate": Value Change {
        (unwired) T27."Image" ("Calibration Tab")
        n228 = event-data() -> ("NewVal"=w468:bool)  [unwired: 1 in]
        n229 = Unbundle By Name(w465) -> ("Stage XYZ Position"=w464:refnum<vi>)
        n230 = property class="Clust (strict)"(reference=w464) -> ("Value"=w463:cluster{"X":sgl, "Y":sgl, "Z":sgl})  [unwired: 1 in, 2 out]
        n231 = Unbundle By Name(w463) -> ("X"=w462:sgl, "Y"=w461:sgl, "Z"=w460:sgl)
        n232 = Equal To 0?(x=w462) -> (x = 0?=w459:bool)
        n233 = Equal To 0?(x=w461) -> (x = 0?=w458:bool)
        n234 = Equal To 0?(x=w460) -> (x = 0?=w457:bool)
        n235 = Compound Arithmetic op=AND(w459, w458, w457) -> (w456:bool)
        n236 = case shown="True" w456 {
          selector: w456 -> [_ w469]
          frame False {
          }
          frame True {
            "Stage Zeroed ?" <- w469
          }
        }
        n237 = case shown="True" w468 {
          tunnel: w467 -> [_ w472]
          tunnel: "Calibration type" -> [_ w471]
          frame False {
          }
          frame True {
            n238 = case shown="True" TRUE {
              tunnel: w472 -> [_ w481]
              tunnel: w471 -> [_ w479]
              frame False {
                n239 = One Button Dialog(message="Please move the bead to a central position and\n'zero' the XYZ stage ") -> ()  [unwired: 1 in, 1 out]
              }
              frame True {
                (unwired) enum16{"X-Y", "Z"}."X-Y" ("Parameter")
                n240 = Bundle By Name(cluster=T39 {"Procedure"=enum."Measure", "Parameter"=enum."XY-X", "Symmetric"=FALSE} ("input cluster"), "Procedure"=ProcedureState."Calibrate", "Parameter"=Control_Plane."XY-X") -> (w475:T39)
                n241 = disable-structure shown="Enabled" {
                  disable-tunnel: [w485 w509] -> w482
                  disable-tunnel: [w484 w508] -> w480
                  disable-tunnel: w479 -> [w483 _]
                  disable-tunnel: "Scaling" ("Message") -> [_ w509]
                  disable-tunnel: w475 -> [_ w508]
                  frame Disabled {
                    n242 = case shown="\"Z-Scaling\"" w483 {
                      tunnel: ["Diffs and Distortion" ("Message") "Magnification" ("Message") "Sums" ("Message") "Scaling" ("Message") "Scaling" ("Message")] -> w485
                      tunnel: [w487 w492 w496 w501 w506] -> w484
                      frame "Offset Differences", Default {
                        n243 = Bundle By Name(cluster=T39 {"Procedure"=enum."Measure", "Parameter"=enum."XY-X", "Symmetric"=FALSE} ("input cluster"), "Procedure"=ProcedureState."Calibrate") -> (w487:T39)
                      }
                      frame "Magnification" {
                        n244 = Bundle By Name(cluster=T39 {"Procedure"=enum."Measure", "Parameter"=enum."XY-X", "Symmetric"=FALSE} ("input cluster"), "Procedure"=ProcedureState."Calibrate") -> (w492:T39)
                      }
                      frame "Offset Sums" {
                        n245 = Bundle By Name(cluster=T39 {"Procedure"=enum."Measure", "Parameter"=enum."XY-X", "Symmetric"=FALSE} ("input cluster"), "Procedure"=ProcedureState."Calibrate") -> (w496:T39)
                      }
                      frame "X-Y Scaling" {
                        n246 = Bundle By Name(cluster=T39 {"Procedure"=enum."Measure", "Parameter"=enum."XY-X", "Symmetric"=FALSE} ("input cluster"), "Procedure"=ProcedureState."Calibrate", "Parameter"=enum16{"X-Y", "Z"}."X-Y") -> (w501:T39)
                      }
                      frame "Z-Scaling" {
                        n247 = Bundle By Name(cluster=T39 {"Procedure"=enum."Measure", "Parameter"=enum."XY-X", "Symmetric"=FALSE} ("input cluster"), "Procedure"=ProcedureState."Calibrate", "Parameter"=enum16{"X-Y", "Z"}."Z") -> (w506:T39)
                      }
                    }
                  }
                  frame Enabled {
                  }
                }
                n248 = call "Enqueue Message.vi"("Message Data"=w480, "Message"=w482, "Queue"=w481) -> ()  [unwired: 7 in, 2 out]
              }
            }
          }
        }
        n249 = property on="Calibration Tab" class="TabCtl (strict)"("Value"=T14."Live Image" ("Calibration Tab")) -> ()  [unwired: 2 in, 2 out]
      }
      event "Sequence": Value Change {
        (unwired) T27."Image" ("Calibration Tab")
        n250 = event-data() -> ("NewVal"=w522:bool)  [unwired: 1 in]
        n251 = Unbundle By Name(w520) -> ("Stage XYZ Position"=w519:refnum<vi>)
        n252 = property class="Clust (strict)"(reference=w519) -> ("Value"=w518:cluster{"X":sgl, "Y":sgl, "Z":sgl})  [unwired: 1 in, 2 out]
        n253 = Unbundle By Name(w518) -> ("X"=w517:sgl, "Y"=w516:sgl, "Z"=w515:sgl)
        n254 = Equal To 0?(x=w517) -> (x = 0?=w514:bool)
        n255 = Equal To 0?(x=w516) -> (x = 0?=w513:bool)
        n256 = Equal To 0?(x=w515) -> (x = 0?=w512:bool)
        n257 = Compound Arithmetic op=AND(w514, w513, w512) -> (w511:bool)
        n258 = case shown="True" w511 {
          selector: w511 -> [_ w523]
          frame False {
          }
          frame True {
            "Stage Zeroed ? 2" <- w523
          }
        }
        n259 = case shown="True" w522 {
          tunnel: w521 -> [_ w525]
          frame False {
          }
          frame True {
            n260 = case shown="True" TRUE {
              tunnel: w525 -> [_ w533]
              frame False {
                n261 = One Button Dialog(message="Please move the bead to a central position and\n'zero' the XYZ stage ") -> ()  [unwired: 1 in, 1 out]
              }
              frame True {
                (unwired) enum16{"X-Y", "Z"}."X-Y" ("Parameter")
                n262 = Bundle By Name(cluster=T39 {"Procedure"=enum."Measure", "Parameter"=enum."XY-X", "Symmetric"=FALSE} ("input cluster"), "Procedure"=ProcedureState."Sequence", "Parameter"=Control_Plane."XY-X") -> (w528:T39)
                n263 = disable-structure shown="Enabled" {
                  disable-tunnel: [w537 w561] -> w534
                  disable-tunnel: [w536 w560] -> w532
                  disable-tunnel: _ -> [w535 _]
                  disable-tunnel: "Scaling" ("Message") -> [_ w561]
                  disable-tunnel: w528 -> [_ w560]
                  frame Disabled {
                    n264 = case shown="\"Z-Scaling\"" w535 {
                      tunnel: ["Diffs and Distortion" ("Message") "Magnification" ("Message") "Sums" ("Message") "Scaling" ("Message") "Scaling" ("Message")] -> w537
                      tunnel: [w539 w544 w548 w553 w558] -> w536
                      frame "Offset Differences", Default {
                        n265 = Bundle By Name(cluster=T39 {"Procedure"=enum."Measure", "Parameter"=enum."XY-X", "Symmetric"=FALSE} ("input cluster"), "Procedure"=ProcedureState."Calibrate") -> (w539:T39)
                      }
                      frame "Magnification" {
                        n266 = Bundle By Name(cluster=T39 {"Procedure"=enum."Measure", "Parameter"=enum."XY-X", "Symmetric"=FALSE} ("input cluster"), "Procedure"=ProcedureState."Calibrate") -> (w544:T39)
                      }
                      frame "Offset Sums" {
                        n267 = Bundle By Name(cluster=T39 {"Procedure"=enum."Measure", "Parameter"=enum."XY-X", "Symmetric"=FALSE} ("input cluster"), "Procedure"=ProcedureState."Calibrate") -> (w548:T39)
                      }
                      frame "X-Y Scaling" {
                        n268 = Bundle By Name(cluster=T39 {"Procedure"=enum."Measure", "Parameter"=enum."XY-X", "Symmetric"=FALSE} ("input cluster"), "Procedure"=ProcedureState."Calibrate", "Parameter"=enum16{"X-Y", "Z"}."X-Y") -> (w553:T39)
                      }
                      frame "Z-Scaling" {
                        n269 = Bundle By Name(cluster=T39 {"Procedure"=enum."Measure", "Parameter"=enum."XY-X", "Symmetric"=FALSE} ("input cluster"), "Procedure"=ProcedureState."Calibrate", "Parameter"=enum16{"X-Y", "Z"}."Z") -> (w558:T39)
                      }
                    }
                  }
                  frame Enabled {
                  }
                }
                n270 = call "Enqueue Message.vi"("Message Data"=w532, "Message"=w534, "Queue"=w533) -> ()  [unwired: 7 in, 2 out]
              }
            }
          }
        }
        n271 = property on="Calibration Tab" class="TabCtl (strict)"("Value"=T14."Live Image" ("Calibration Tab")) -> ()  [unwired: 2 in, 2 out]
      }
      event "Test": Value Change {
        n272 = event-data() -> ("NewVal"=w574:bool)  [unwired: 1 in]
        n273 = Unbundle By Name(w563) -> ("Stage XYZ Position"=w571:refnum<vi>)
        n274 = property class="Clust (strict)"(reference=w571) -> ("Value"=w570:cluster{"X":sgl, "Y":sgl, "Z":sgl})  [unwired: 1 in, 2 out]
        n275 = Unbundle By Name(w570) -> ("X"=w569:sgl, "Y"=w568:sgl, "Z"=w567:sgl)
        n276 = Equal To 0?(x=w569) -> (x = 0?=w566:bool)
        n277 = Equal To 0?(x=w568) -> (x = 0?=w565:bool)
        n278 = Equal To 0?(x=w567) -> (x = 0?=w564:bool)
        n279 = Compound Arithmetic op=OR(w566, w565, w564) -> (w562:bool)
        n280 = case shown="True" w574 {
          tunnel: w573 -> [_ w576]
          tunnel: "Calibration test type" -> [_ w577]
          tunnel: w562 -> [_ w575]
          frame False {
          }
          frame True {
            n281 = case shown="True" w575 {
              tunnel: w577 -> [_ w580]
              tunnel: w576 -> [_ w579]
              frame False {
                n282 = One Button Dialog(message="Please move the bead to a central position and\n'zero' the XYZ stage ") -> ()  [unwired: 1 in, 1 out]
              }
              frame True {
                n283 = case shown="\"Dwell Times\"" w580 {
                  tunnel: ["Sums" ("Message") "Diffs and Distortion" ("Message") "Dwell Times" ("Message")] -> w582
                  tunnel: [w584 w589 w593] -> w581
                  frame "Sums", Default {
                    n284 = Bundle By Name(cluster=T39 {"Procedure"=enum."Measure", "Parameter"=enum."XY-X", "Symmetric"=FALSE} ("input cluster"), "Procedure"=ProcedureState."Test") -> (w584:T39)
                  }
                  frame "Diffs and Distortion" {
                    n285 = Bundle By Name(cluster=T39 {"Procedure"=enum."Measure", "Parameter"=enum."XY-X", "Symmetric"=FALSE} ("input cluster"), "Procedure"=ProcedureState."Test") -> (w589:T39)
                  }
                  frame "Dwell Times" {
                    n286 = Bundle By Name(cluster=T39 {"Procedure"=enum."Measure", "Parameter"=enum."XY-X", "Symmetric"=FALSE} ("input cluster"), "Procedure"=ProcedureState."Test") -> (w593:T39)
                  }
                }
                n287 = call "Enqueue Message.vi"("Message Data"=w581, "Message"=w582, "Queue"=w579) -> ()  [unwired: 7 in, 2 out]
              }
            }
          }
        }
      }
      event "Testing Range (Norm)_min", "Testing Range (Norm)_max", "Auto Focus", "Search_max", "Search_min", "Calibration_max", "Calibration_min", "auto-set pockel", "Pockels Cell Value for pointing mode": Value Change {
        n288 = event-data() -> ()  [unwired: 1 in, 6 out]
      }
      event "Measure PSF": Value Change {
        n289 = event-data() -> ("NewVal"=w595:bool)  [unwired: 1 in]
        n290 = case shown="True" w595 {
          tunnel: w596 -> [_ w600]
          frame False {
          }
          frame True {
            n291 = Bundle By Name(cluster=T39 {"Procedure"=enum."Measure", "Parameter"=enum."XY-X", "Symmetric"=FALSE} ("input cluster"), "Procedure"=ProcedureState."Measure") -> (w599:T39)
            n292 = call "Enqueue Message.vi"("Message Data"=w599, "Message"="Measure PSF", "Queue"=w600) -> ()  [unwired: 7 in, 2 out]
          }
        }
      }
      event "Reload": Value Change {
        n293 = event-data() -> ("NewVal"=w605:bool)  [unwired: 1 in, 5 out]
        n294 = case shown="True" w605 {
          tunnel: "Current Calibration Parameters" -> [_ w629]
          tunnel: "Current Objective" -> [_ _]
          tunnel: [errorcluster {"status"=FALSE, "code"=0, "source"=""} ("error out") w614] -> w602
          frame False {
          }
          frame True {
            (unwired) T27."Image" ("Calibration Tab")
            n295 = call "fgv_calibration_config.vi"("Cal config ops"=T23."Load from file") -> ("error out"=w619:errorcluster, "Config file path"=w615:path, "Config cluster OUT"=w616:T28)  [unwired: 8 in]
            n296 = control-ref of="Objectives"() -> (w618:refnum<vi>)
            n297 = Open/Create/Replace File(file path (use dialog)=w615) -> (refnum out=w625:refnum<file>, error out=w624:errorcluster)  [unwired: 5 in, 1 out]
            n298 = property on="Calibration.ini Path" class="Path"("Value"=w615) -> ()  [unwired: 2 in, 2 out]
            n299 = call "Update fgv objectives.vi"("error in (no error)"=w619, "Config cluster IN"=w616) -> ("Available Objectives"=w623:string[], "Current Objective"=w622:string)  [unwired: 7 in, 1 out]
            n300 = Read from Text File(file (use dialog)=w625, error in=w624) -> (refnum out=w626:refnum<file>, text=w617:string, error out=w627:errorcluster)  [unwired: 2 in, 1 out]
            n301 = call "Update Objective tree.vi"("Visible Items:Column Headers Visible"=TRUE, "error in (no error)"=w619, "Column Header Strings[]"=string[] ["Item", "Value"], "Config cluster IN"=w616, "TreeControl in"=w618) -> ("error out"=w614:errorcluster)  [unwired: 6 in]
            n302 = property on="Objective" class="CmbBox (strict)"("Strings[]"=w623, "Value"=w622) -> ()  [unwired: 2 in, 2 out]
            n303 = Close File(refnum=w626, error in=w627) -> ()  [unwired: 2 out]
            n304 = property on="Calibration.ini" class="Str"("Value"=w617) -> ()  [unwired: 2 in, 2 out]
            n305 = call "Update Objective calibration data.vi"("Config cluster OUT"=w616, "Current Calibration Parameters in"=w629) -> ("Current Calibration Parameters out"=w612:T10)  [unwired: 8 in, 1 out]
            n306 = Unbundle By Name(w612) -> ("Sum X"=w611:dbl, "Sum Y"=w610:dbl, "Diff X"=w609:dbl, "Diff Y"=w608:dbl, "Distortion Correction"=w607:dbl)
            n307 = local write "Current Calibration Parameters"(w612) -> ()
            n308 = property on="Calibration Tab" class="TabCtl (strict)"("Value"=T14."Live Image" ("Calibration Tab")) -> ()  [unwired: 2 in, 2 out]
            n309 = local write "Sum X"(w611) -> ()
            n310 = local write "Sum Y"(w610) -> ()
            n311 = local write "Diff X"(w609) -> ()
            n312 = local write "Diff Y"(w608) -> ()
            n313 = local write "Distortion Corr."(w607) -> ()
          }
        }
      }
      event Value Change {
        n314 = event-data() -> ("OldVal"=w632:T10, "NewVal"=w630:T10)  [unwired: 1 in, 4 out]
        n315 = Not Equal?(x=w632, y=w630) -> (x != y?=w631:bool)
        n316 = case shown="True" w631 {
          tunnel: w630 -> [_ w636]
          frame False {
          }
          frame True {
            n317 = global read "General Globals.vi" "Objective"() -> (w637:string)
            n318 = call "Update_Matlab_for_calib.vi"("Current Calibration Parameters"=w636) -> ("error out"=w635:errorcluster)  [unwired: 10 in]
            n319 = call "Force update objective calibration settings .vi"("Current Calibration Parameters"=w636, "Current Objective"=w637) -> ("error out"=w634:errorcluster)  [unwired: 9 in]
            n320 = Merge Errors(w635, w634) -> (w633:errorcluster)
            n321 = flat-sequence {
              tunnel: w633 -> [w641]
              tunnel: [w640] -> w639
              tunnel: [w644] -> w638
              tunnel: w639 -> [w644]
              tunnel: w638 -> [w647]
              tunnel: [w646] -> _
              frame #0 {
                n322 = call "Fire User Event - Next State.vi"("Error In"=w641, "\"UI Handler loop\" case to execute"=Top_level_VI_states."Live Imaging-STOP" ("event data / imaging mode")) -> ("Error Out"=w640:errorcluster)  [unwired: 9 in]
              }
              frame #1 {
                n323 = Wait (ms)(milliseconds to wait=u32 1000) -> ()  [unwired: 1 out]
              }
              frame #2 {
                n324 = call "Fire User Event - Next State.vi"("Error In"=w647, "\"UI Handler loop\" case to execute"=Top_level_VI_states."Live Imaging-START" ("event data / imaging mode")) -> ("Error Out"=w646:errorcluster)  [unwired: 9 in]
              }
            }
          }
        }
      }
      event Value Change {
        n325 = event-data() -> ()  [unwired: 1 in, 6 out]
        n326 = property on="Current Calibration Parameters" class="Clust (strict)"() -> ("Value"=w658:T10)  [unwired: 2 in, 2 out]
        n327 = Bundle By Name(cluster=w658, "Sum X"="Sum X", "Sum Y"="Sum Y", "Diff X"="Diff X", "Diff Y"="Diff Y", "Distortion Correction"="Distortion Corr.") -> (w656:T10)
        n328 = property on="Current Calibration Parameters" class="Clust (strict)"("Value"=w656) -> (error out=w657:errorcluster)  [unwired: 2 in, 1 out]
        n329 = call "Update_Matlab_for_calib.vi"("error in (no error)"=w657, "Current Calibration Parameters"=w656) -> ("error out"=w653:errorcluster)  [unwired: 9 in]
        n330 = flat-sequence {
          tunnel: w653 -> [w660]
          tunnel: [w659] -> w655
          tunnel: [w663] -> w654
          tunnel: w655 -> [w663]
          tunnel: w654 -> [w666]
          tunnel: [w665] -> _
          frame #0 {
            n331 = call "Fire User Event - Next State.vi"("Error In"=w660, "\"UI Handler loop\" case to execute"=Top_level_VI_states."Live Imaging-STOP" ("event data / imaging mode")) -> ("Error Out"=w659:errorcluster)  [unwired: 9 in]
          }
          frame #1 {
            n332 = Wait (ms)(milliseconds to wait=u32 200) -> ()  [unwired: 1 out]
          }
          frame #2 {
            n333 = call "Fire User Event - Next State.vi"("Error In"=w666, "\"UI Handler loop\" case to execute"=Top_level_VI_states."Live Imaging-START" ("event data / imaging mode")) -> ("Error Out"=w665:errorcluster)  [unwired: 9 in]
          }
        }
      }
      event "Visible(Grid)", "Grid Lines": Value Change {
        n334 = event-data() -> ()  [unwired: 1 in, 1 out]
        n335 = case shown="False" "Visible(Grid)" {
          frame False {
            n336 = local read "Image"() -> (w669:T5)
            n337 = call "IMAQ Clear Overlay"("Image"=w669) -> ("Image Out"=w668:T5)  [unwired: 9 in, 1 out]
            n338 = local write "Image"(w668) -> ()
          }
          frame True {
            n339 = local read "Image"() -> (w676:T5)
            n340 = property class="IMAQImage"(reference=w676) -> (reference out=w673:T5, error out=w672:errorcluster, "ImageSize"=w675:cluster{"x":i32, "y":i32})  [unwired: 1 in]
            n341 = Unbundle By Name(w675) -> ("x"=w670:i32)
            n342 = Not Equal To 0?(x=w670) -> (x != 0?=w674:bool)
            n343 = case shown="True" w674 {
              tunnel: w673 -> [_ w680]
              tunnel: w672 -> [_ w679]
              tunnel: "Grid Lines" -> [_ w677]
              frame False {
              }
              frame True {
                n344 = call "Draw_Grid.vi"("error in (no error)"=w679, "Grid Lines"=w677, "Image In"=w680) -> ("Image Out"=w681:T5)  [unwired: 7 in, 1 out]
                n345 = local write "Visible(Grid)"(TRUE ("Visible(Grid)")) -> ()
                n346 = local write "Image"(w681) -> ()
              }
            }
          }
        }
      }
      event "CH1", "CH2": Value Change {
        n347 = event-data() -> ("CtlRef"=w684:refnum<vi>, "NewVal"=w685:bool)  [unwired: 1 in, 4 out]
        n348 = property class="Bool (strict)"(reference=w684) -> ("Label.Text"=w682:string)  [unwired: 1 in, 2 out]
        n349 = case shown="\"CH2\"" w682 {
          tunnel: w685 -> [w688 w715]
          tunnel: [w687 w714] -> w683
          tunnel: w682 -> [w686 w713]
          frame "CH2" {
            n350 = disable-structure shown="Disabled" {
              disable-tunnel: w688 -> [w691 _]
              disable-tunnel: [w690 _] -> w687
              disable-tunnel: w686 -> [w689 _]
              frame Disabled {
                n351 = case shown="True" w691 {
                  tunnel: [w694 w698] -> w690
                  tunnel: w689 -> [w693 w697]
                  frame False {
                    n352 = local read "Core Image"() -> (w696:T5)
                    n353 = Build Array(w693) -> (w692:string[])
                    n354 = call "IMAQ Clear Overlay"("Groups"=w692, "Image"=w696) -> ("error out"=w694:errorcluster, "Image Out"=w695:T5)  [unwired: 8 in]
                    n355 = local write "Core Image"(w695) -> ()
                  }
                  frame True {
                    n356 = local read "Core Image"() -> (w699:T5)
                    n357 = property class="IMAQImage"(reference=w699) -> (reference out=w702:T5, error out=w701:errorcluster, "ImageSize"=w704:cluster{"x":i32, "y":i32})  [unwired: 1 in]
                    n358 = Unbundle By Name(w704) -> ("x"=w700:i32)
                    n359 = Not Equal To 0?(x=w700) -> (x != 0?=w703:bool)
                    n360 = case shown="True" w703 {
                      tunnel: w702 -> [_ w712]
                      tunnel: w701 -> [w705 w711]
                      tunnel: [w705 w707] -> w698
                      tunnel: w697 -> [_ w706]
                      frame False {
                      }
                      frame True {
                        n361 = call "Draw_fixed_grid.vi"("Grid Line Color"=u32 16776960, "error in (no error)"=w711, "Grid name"=w706, "Grid Lines"=u32 2, "Image In"=w712) -> ("error out"=w707:errorcluster, "Image Out"=w709:T5)  [unwired: 5 in]
                        n362 = local write "Core Image"(w709) -> ()
                      }
                    }
                  }
                }
              }
              frame Enabled {
              }
            }
          }
          frame "CH1", Default {
            n363 = case shown="False" w715 {
              tunnel: [w718 w722] -> w714
              tunnel: w713 -> [w717 w721]
              frame False {
                n364 = Build Array(w717) -> (w716:string[])
                n365 = local read "Image"() -> (w720:T5)
                n366 = call "IMAQ Clear Overlay"("Groups"=w716, "Image"=w720) -> ("error out"=w718:errorcluster, "Image Out"=w719:T5)  [unwired: 8 in]
                n367 = local write "Image"(w719) -> ()
              }
              frame True {
                n368 = local read "Image"() -> (w728:T5)
                n369 = property class="IMAQImage"(reference=w728) -> (reference out=w725:T5, error out=w724:errorcluster, "ImageSize"=w727:cluster{"x":i32, "y":i32})  [unwired: 1 in]
                n370 = Unbundle By Name(w727) -> ("x"=w723:i32)
                n371 = Not Equal To 0?(x=w723) -> (x != 0?=w726:bool)
                n372 = case shown="True" w726 {
                  tunnel: w725 -> [_ w734]
                  tunnel: w724 -> [w729 w733]
                  tunnel: [w729 w731] -> w722
                  tunnel: w721 -> [_ w730]
                  frame False {
                  }
                  frame True {
                    n373 = call "Draw_fixed_grid.vi"("error in (no error)"=w733, "Grid name"=w730, "Grid Lines"=u32 2, "Image In"=w734) -> ("error out"=w731:errorcluster, "Image Out"=w735:T5)  [unwired: 6 in]
                    n374 = local write "Image"(w735) -> ()
                  }
                }
              }
            }
          }
        }
        "error out 10" <- w683
      }
      event "Live Image intensity": Value Change {
        n375 = event-data() -> ("NewVal"=w737:cluster{i16, i16})  [unwired: 1 in, 5 out]
        n376 = control-ref of="Image"() -> (w736:refnum<vi>)
        n377 = call "16 bit display mapping.vi"("16 bit display mapping"=w737, "Image Display"=w736) -> ()  [unwired: 8 in, 2 out]
      }
      event "Intensity Graph colour palette": Value Change {
        n378 = event-data() -> ("NewVal"=w738:cluster{dbl, "Color Box":u32}[])  [unwired: 1 in, 5 out]
        n379 = property on="Intensity" class="IntGraph (strict)"("ZScale.MarkerVals[]"=w738) -> ()  [unwired: 2 in, 2 out]
      }
      event "core Intensity Graph colour palette": Value Change {
        n380 = event-data() -> ()  [unwired: 1 in, 6 out]
        n381 = property on="Core Intensity" class="IntGraph (strict)"("ZScale.MarkerVals[]"="core Intensity Graph colour palette") -> ()  [unwired: 2 in, 2 out]
      }
      event "Add reference": Value Change {
        n382 = event-data() -> ()  [unwired: 1 in, 6 out]
        n383 = local read "AOLZ"() -> (w759:sgl)
        n384 = local read "Y Centre"() -> (w757:sgl)
        n385 = local read "X Centre"() -> (w758:sgl)
        n386 = Unbundle By Name(w741) -> ("Z"=w756:sgl, "X"=w755:sgl, "Y"=w754:sgl)
        n387 = Build Array(w759, w758, w757, w756, w755, w754) -> (w744:sgl[])
        n388 = call "fgv_pos_reference.vi"("State"=enum16{"Initialise", "Write", "Read", "Clear"}."Write", "Pos ref in"=w744) -> ("error in (no error)"=w752:errorcluster, "Pos Value"=w743:sgl)  [unwired: 7 in, 1 out]
        n389 = Insert Into Array(array=w744, index=0, new element=w743) -> (w742:sgl[])
        n390 = call "fgv_calibrationPos_LBVals.vi"("ACtions"=enum16{"Initialise", "Get", "Set"}."Get") -> ("Calibration Pos LBVals  OUT"=w749:string[][])  [unwired: 9 in, 1 out]
        n391 = Number To Fractional String(number=w742, precision (6)=i16 2) -> (F-format string=w748:string[])  [unwired: 2 in]
        n392 = Build Array (concatenate)(w749, w748) -> (w746:string[][])
        n393 = call "fgv_calibrationPos_LBVals.vi"("ACtions"=enum16{"Initialise", "Get", "Set"}."Set", "Calibration Pos LBVals IN"=w746) -> ()  [unwired: 8 in, 2 out]
        n394 = property on="Saved Pos" class="MCListbox (strict)"(error in=w752, "ItemNames"=w746) -> ()  [unwired: 1 in, 2 out]
      }
      event "Clear selected": Value Change {
        n395 = event-data() -> ()  [unwired: 1 in, 6 out]
        n396 = call "fgv_calibrationPos_LBVals.vi"("ACtions"=enum16{"Initialise", "Get", "Set"}."Get", "error in (no error)"=w763) -> ("error out"=w762:errorcluster, "Calibration Pos LBVals  OUT"=w765:string[][])  [unwired: 8 in]
        n397 = for {
          tunnel: "Saved Pos" -> [w769] mode=indexing
          shift-right: [w773] -> w760
          shift-left: w765 -> [w774]
          i -> [w771]
          n398 = Increment(x=w771) -> (x+1=w768:i32)
          n399 = Subtract(x=w769, y=w768) -> (x-y=w770:i32)
          n400 = Delete From Array(array=w774, length=0, index (row)=w770) -> (array with subset deleted=w773:string[][])  [unwired: 1 in, 1 out]
        }
        n401 = property on="Saved Pos" class="MCListbox (strict)"("ItemNames"=w760) -> ()  [unwired: 2 in, 2 out]
        n402 = call "fgv_calibrationPos_LBVals.vi"("ACtions"=enum16{"Initialise", "Get", "Set"}."Set", "error in (no error)"=w762, "Calibration Pos LBVals IN"=w760) -> ("error out"=w761:errorcluster)  [unwired: 7 in, 1 out]
      }
      event "Clear all": Value Change {
        n403 = event-data() -> ()  [unwired: 1 in, 6 out]
        n404 = call "fgv_pos_reference.vi"("State"=enum16{"Initialise", "Write", "Read", "Clear"}."Initialise") -> ("error in (no error)"=w775:errorcluster)  [unwired: 8 in, 2 out]
        n405 = property on="Saved Pos" class="MCListbox (strict)"(error in=w775, "ItemNames"=string[][] [] ("Item Names")) -> ()  [unwired: 1 in, 2 out]
      }
      event "Saved Pos": Edit Cell {
        n406 = event-data() -> ()  [unwired: 1 in, 6 out]
        n407 = property on="Saved Pos" class="MCListbox (strict)"() -> ("ItemNames"=w779:string[][])  [unwired: 2 in, 2 out]
        n408 = call "fgv_calibrationPos_LBVals.vi"("ACtions"=enum16{"Initialise", "Get", "Set"}."Set", "Calibration Pos LBVals IN"=w779) -> ()  [unwired: 8 in, 2 out]
      }
      event "Core extraction size", "X offset", "Y offset": Value Change {
        n409 = event-data() -> ()  [unwired: 1 in, 6 out]
        n410 = disable-structure shown="Enabled" {
          frame Disabled {
            n411 = local read "Y Res."() -> ()  [unwired: 1 out]
            n412 = local read "X Res."() -> ()  [unwired: 1 out]
            n413 = Open Python Session(python version="3.6" ("Python version")) -> (session out=w782:refnum<k35>)  [unwired: 2 in, 1 out]
            n414 = node(w782, path "C:/LocalSVNSCC/local_copy_ml/Configuration code/Calibration/ToolBox/Python_scripts" ("module path"), "core2didx.py" ("function name")) -> ()  [unwired: 3 in, 4 out]
            n415 = Close Python Session() -> ()  [unwired: 2 in, 1 out]
          }
          frame Enabled {
          }
        }
      }
      event "Save to file": Value Change {
        n416 = event-data() -> ()  [unwired: 1 in, 6 out]
        n417 = property on="Saved Pos" class="MCListbox (strict)"() -> ("ItemNames"=w784:string[][])  [unwired: 2 in, 2 out]
        n418 = Format Date/Time String(time format string (%c)="%d%m%Y_%H%M%S") -> (date/time string=w796:string)  [unwired: 2 in]
        n419 = Concatenate Strings("pos_data_", w796, ".csv" ("string")) -> (w792:string)
        n420 = Build Path(base path=path "C:/Support Files/Calibration data", name or relative path=w792) -> (appended path=w794:path)
        n421 = Array To Spreadsheet String(delimiter (Tab)=",", array=w784, 3:"%s" ("format string")) -> (spreadsheet string=w789:string)
        n422 = Open/Create/Replace File(file path (use dialog)=w794, error in=errorcluster {"status"=FALSE, "code"=0, "source"=""}, operation (0:open)=T44."open or create") -> (refnum out=w791:refnum<file>, error out=w790:errorcluster)  [unwired: 3 in, 1 out]
        n423 = Write to Text File(file (use dialog)=w791, text=w789, error in=w790) -> (refnum out=w787:refnum<file>, error out=w788:errorcluster)  [unwired: 1 in, 1 out]
        n424 = Close File(refnum=w787, error in=w788) -> (error out=→"error out 5":errorcluster)  [unwired: 1 out]
      }
      event "Zero Stage": Value Change {
        n425 = event-data() -> ()  [unwired: 1 in, 6 out]
        n426 = Bundle By Name(cluster=T42 {"Command"=enum."Initialize", "Channel"="", "X"=0.0, "Y"=0.0, "Z"=0.0, "Speed"=0, "Zero"=FALSE, "Use acknowledgement?"=FALSE} ("XYZ Stage data to queue"), "Channel"=T41 "All") -> (w805:T42)
        n427 = call "XYZ Stage-Command request module.vi"("Command"=XYZ_stage_states."Reset Axis", "XYZ Stage data to queue"=w805) -> ()  [unwired: 5 in, 5 out]
      }
      event "Core image": Value Change {
        n428 = event-data() -> ("NewVal"=w807:cluster{"Numeric":dbl, "Numeric":dbl})  [unwired: 1 in, 5 out]
        n429 = control-ref of="Core Image"() -> (w806:refnum<vi>)
        n430 = call "16 bit display mapping.vi"("16 bit display mapping"=w807, "Image Display"=w806) -> ()  [unwired: 8 in, 2 out]
      }
      event "Freeze Image": Value Change {
        n431 = event-data() -> ()  [unwired: 1 in, 6 out]
        n432 = disable-structure shown="Disabled" {
          disable-tunnel: w808 -> [w811 _]
          frame Disabled {
            n433 = local read "Current Calibration Parameters"() -> (w813:T10)
            n434 = local read "Image"() -> (w814:T5)
            n435 = call "fgv_AOL_Globals Read.vi"() -> ("AOL_Globals"=w812:T45)  [unwired: 9 in, 2 out]
            n436 = call "Image and data to image buffer FGV.vi"("Current Calibration Parameters"=w813, "AOL_Globals"=w812, "Stage XYZ Position"=w811, "Refnum in"=w814) -> ("LB data full"=→"LB data full":string[][], "LB data"=→"LB data":string[][])  [unwired: 4 in, 2 out]
          }
          frame Enabled {
          }
        }
      }
      event "Freeze Core Image": Value Change {
        w817 = T18 1 items=["Grayscale (U8)", "Grayscale (I16)", "Grayscale (SGL)", "Complex (CSG)", "RGB (U32)", "HSL (U32)", "RGB (U64)", "Grayscale (U16)"] ("Image Type")
        n437 = event-data() -> ()  [unwired: 1 in, 6 out]
        n438 = local read "Core Image"() -> (w816:T5)
        n439 = call "IMAQ Create"("Image Name"="Temp Buffer 4", "Image Type"=w817) -> ("New Image"=w819:T5)  [unwired: 3 in, 1 out]
        n440 = call "IMAQ Copy"("Image Dst"=w819, "Image Src"=w816) -> ("Image Dst Out"=→"Core Image frozen":T5)  [unwired: 4 in, 1 out]
      }
      event "Measure": Value Change {
        w821 = errorcluster {"status"=FALSE, "code"=0, "source"=""} ("error in (no error)")
        n441 = event-data() -> ()  [unwired: 1 in, 6 out]
        n442 = local read "Frozen image"() -> (w822:T5)
        n443 = call "fgv buffer image references.vi"("Image Reference IN"=w822, "Actions"=data_and_image_buffer_fgv_actions."Add Image to buffer", "error in (no error)"=w821) -> ()  [unwired: 6 in, 7 out]
        n444 = disable-structure shown="Disabled" {
          disable-tunnel: w821 -> [w826 _]
          disable-tunnel: [w825 _] -> w823
          disable-tunnel: w822 -> [w824 _]
          frame Disabled {
            n445 = call "Measure distance v2.vi"("error in (no error)"=w826, "Input image"=w824) -> ("error out"=w825:errorcluster)  [unwired: 9 in]
          }
          frame Enabled {
          }
        }
        "error out 7" <- w823
      }
      event "Frozen Image intensity": Value Change {
        n446 = event-data() -> ("NewVal"=w827:cluster{i16, i16})  [unwired: 1 in, 5 out]
        n447 = control-ref of="Frozen image"() -> (w828:refnum<vi>)
        n448 = call "16 bit display mapping.vi"("16 bit display mapping"=w827, "Image Display"=w828) -> ()  [unwired: 8 in, 2 out]
      }
      event "Frozen core image intensity": Value Change {
        n449 = event-data() -> ("NewVal"=w829:cluster{"Numeric":dbl, "Numeric":dbl})  [unwired: 1 in, 5 out]
        n450 = control-ref of="Frozen image"() -> (w830:refnum<vi>)
        n451 = call "16 bit display mapping.vi"("16 bit display mapping"=w829, "Image Display"=w830) -> ()  [unwired: 8 in, 2 out]
      }
      event "Overlay\ncore": Value Change {
        n452 = event-data() -> ()  [unwired: 1 in, 6 out]
        n453 = disable-structure shown="Disabled" {
          frame Disabled {
            n454 = local read "Image"() -> ()  [unwired: 1 out]
          }
          frame Enabled {
          }
        }
      }
      event "Sums Incr", "Diffs Incr", "DC Incr": Value Change {
        n455 = event-data() -> ("CtlRef"=w832:refnum<vi>)  [unwired: 1 in, 5 out]
        n456 = property class="DigNum (strict)"(reference=w832) -> ("Label.Text"=w831:string)  [unwired: 1 in, 2 out]
        n457 = case shown="Default" w831 {
          frame Default {
            "String" <- "incr update failed" ("String")
          }
          frame "Diffs Incr" {
            n458 = control-ref of="Diff Y"() -> (w835:refnum<vi>)
            n459 = control-ref of="Diff X"() -> (w836:refnum<vi>)
            n460 = property class="DigNum (strict)"(reference=w836, "Increment"="Diffs Incr") -> ()  [unwired: 1 in, 2 out]
            n461 = property class="DigNum (strict)"(reference=w835, "Increment"="Diffs Incr") -> ()  [unwired: 1 in, 2 out]
          }
          frame "Sums Incr" {
            n462 = control-ref of="Sum Y"() -> (w838:refnum<vi>)
            n463 = control-ref of="Sum X"() -> (w839:refnum<vi>)
            n464 = property class="DigNum (strict)"(reference=w839, "Increment"="Sums Incr") -> ()  [unwired: 1 in, 2 out]
            n465 = property class="DigNum (strict)"(reference=w838, "Increment"="Sums Incr") -> ()  [unwired: 1 in, 2 out]
          }
          frame "DC Incr" {
            n466 = control-ref of="Distortion Corr."() -> (w840:refnum<vi>)
            n467 = property class="DigNum (strict)"(reference=w840, "Increment"="DC Incr") -> ()  [unwired: 1 in, 2 out]
          }
        }
      }
      event "Snap save": Value Change {
        n468 = event-data() -> ()  [unwired: 1 in, 6 out]
        n469 = local read "Frozen image"() -> (w843:T5)
        n470 = call "SaveImage_single.vi"("base path"=path "C:/Support Files/Calibration data", "Image Src A"=w843) -> ()  [unwired: 9 in, 1 out]
      }
      event "Incr": Value Change {
        (unwired) string[] ["Sum X", "Sum Y", "Diff X", "Diff Y", "Distortion Correction", "Z_norm to um_scaling", "X_norm to um_scaling", "Samples to Wait after Trigger", "Slip Cycle"] ("Array 2")
        (unwired) string[] ["Sum X", "Sum Y", "Diff X", "Diff Y", "Distortion Correction"] ("Array 2")
        n471 = event-data() -> ()  [unwired: 1 in, 6 out]
        n472 = control-ref of="Current Calibration Parameters"() -> (w846:refnum<vi>)
        n473 = property class="Clust (strict)"(reference=w846) -> ("Controls[]"=w845:refnum<vi>[])  [unwired: 1 in, 2 out]
        n474 = for {
          tunnel: w845 -> [w850] mode=indexing
          tunnel: "Incr" -> [w847]
          n475 = control-ref of="sample dtype"() -> (w848:refnum<vi>)
          n476 = To More Specific Class(target class=w848, reference=w850) -> (specific class reference=w849:refnum<vi>)  [unwired: 1 in, 1 out]
          n477 = property class="DigNum (strict)"(reference=w849, "Increment"=w847) -> ()  [unwired: 1 in, 2 out]
        }
      }
    }
  }
  n478 = while {
    tunnel: w42 -> [w858]
    tunnel: w41 -> [w854]
    tunnel: w39 -> [_]
    tunnel: [w851] -> w26
    stop <- w851 stop-if-true
    n479 = call "Dequeue Message.vi"("Error In"=w854, "timeout in ms (-1)"=10, "Message Queue"=w858) -> ("Error Out"=w853:errorcluster, "Message Data"=w856:variant, "Message"=w857:string)  [unwired: 4 in, 2 out]
    n480 = case shown="\"Scaling\"" w857 {
      tunnel: w856 -> [_ _ _ w870 w879 w904 w908 w915 w925]
      tunnel: T39 {"Procedure"=enum."Measure", "Parameter"=enum."XY-X", "Symmetric"=FALSE} ("input cluster") -> [_ _ _ w869 w880 w903 w909 w914 w923]
      tunnel: w853 -> [_ w860 _ _ w877 _ w907 w916 _]
      tunnel: [w859 _ _ _ _ _ _ _ _] -> w851
      frame Default {
        n481 = local read "Stop_Ind"() -> (w859:bool)
      }
      frame "Exit" {
        n482 = disable-structure shown="Enabled" {
          disable-tunnel: [w864 w868] -> w861
          disable-tunnel: w860 -> [w862 w868]
          frame Disabled {
            n483 = global read "gl_Queues.vi" "UI queue name"() -> (w863:string)
            n484 = call "Obtain Message Queue.vi"("error in (no error)"=w862, "Queue name"=w863) -> ("error out"=w867:errorcluster, "Message Queue"=w866:refnum<queue>)  [unwired: 8 in]
            n485 = call "Enqueue Message.vi"("error in (no error)"=w867, "Message"="Unload subpanel", "Queue"=w866) -> ("error out"=w864:errorcluster)  [unwired: 7 in, 1 out]
          }
          frame Enabled {
          }
        }
        n486 = call <vilib>:"Simple Error Handler.vi"("error in (no error)"=w861) -> ()  [unwired: 4 in, 5 out]
      }
      frame "Initialize" {
      }
      frame "Measure PSF" {
        n487 = Variant To Data(type=w869, Variant=w870) -> (data=w871:T39)  [unwired: 1 in, 1 out]
        n488 = Unbundle By Name(w871) -> ()  [unwired: 1 out]
      }
      frame "Scaling" {
        n489 = Variant To Data(error in=w877, type=w880, Variant=w879) -> (data=w876:T39, error out=w878:errorcluster)
        n490 = local read "Signal Channel"() -> (w874:enum16{"Red", "Green"})
        n491 = local read "Motor Z values"() -> (w873:i32[])
        n492 = local read "AOL Z values"() -> (w872:i32[])
        n493 = disable-structure shown="Disabled" {
          disable-tunnel: w876 -> [w895 _]
          disable-tunnel: w878 -> [w894 _]
          frame Disabled {
            n494 = Unbundle By Name(w895) -> ("Parameter"=w890:T38)
            n495 = call "Calibrate_AOL XYZ.vi"("error in (no error)"=w894, "Stage Control"=w890) -> ("norm_to_um_scaling"=w891:dbl)  [unwired: 8 in, 1 out]
            n496 = case shown="\"XY-X\", Default" w890 {
              tunnel: [w898 w901] -> w893
              tunnel: T10 {"Sum X"=0.0, "Sum Y"=0.0, "Diff X"=0.0, "Diff Y"=0.0, "Distortion Correction"=0.0, "Z_norm to um_scaling"=0.0, "X_norm to um_scaling"=0.0, "Samples to Wait after Trigger"=0.0, "Slip Cycle"=0.0} ("Current Calibration Parameters") -> [w897 w900]
              tunnel: w891 -> [w896 w899]
              frame "Z" {
                n497 = Bundle By Name(cluster=w897, "Z_norm to um_scaling"=w896) -> (w898:T10)
              }
              frame "XY-X", Default {
                n498 = Bundle By Name(cluster=w900, "X_norm to um_scaling"=w899) -> (w901:T10)
              }
            }
            n499 = local write "Current Calibration Parameters"(w893) -> ()
          }
          frame Enabled {
          }
        }
        n500 = Unbundle By Name(w876) -> ("Procedure"=w875:T12)
        n501 = case shown="\"Sequence\"" w875 {
          tunnel: w874 -> [_ w886 w889]
          tunnel: w873 -> [_ w885 _]
          tunnel: w872 -> [_ w884 _]
          frame "Measure", Default {
          }
          frame "Sequence" {
            w882 = T18 1 items=["Grayscale (U8)", "Grayscale (I16)", "Grayscale (SGL)", "Complex (CSG)", "RGB (U32)", "HSL (U32)", "RGB (U64)", "Grayscale (U16)"] ("Image Type")
            n502 = call "Get frame sequence.vi"("Signal Channel"=w886, "AOL Z values"=w884, "Motor Z values"=w885) -> ("Array"=w883:T5[])  [unwired: 7 in, 1 out]
            "Array" <- w883
            n503 = call "MaxZ from Image array.vi"("Image Type"=w882, "Array"=w883) -> ("Image 2"=w881:T5)  [unwired: 8 in, 1 out]
            n504 = local write "Image"(w881) -> ()
          }
          frame "Calibrate" {
            n505 = call "Get single frame.vi"("Signal Channel"=w889) -> ("Image"=w888:T5)  [unwired: 9 in, 1 out]
            n506 = call "IMAQ ImageToArray"("Image"=w888) -> ("Image Pixels (I16)"=→"Image Pixels (I16)" →"Intensity Graph":i16[][])  [unwired: 3 in, 4 out]
            n507 = local write "Image"(w888) -> ()
          }
        }
      }
      frame "Sums" {
        n508 = Variant To Data(type=w903, Variant=w904) -> (data=w905:T39)  [unwired: 1 in, 1 out]
        n509 = Unbundle By Name(w905) -> ("Procedure"=w902:T12)
        "Procedure" <- w902
        n510 = case shown="\"Test\", Default" w902 {
          frame "Test", Default {
          }
          frame "Calibrate" {
            n511 = local read "Signal Channel"() -> (w906:enum16{"Red", "Green"})
            n512 = call "Calibrate_Sums.vi"("Signal Channel"=w906) -> ()  [unwired: 8 in, 3 out]
          }
        }
      }
      frame "Diffs and Distortion" {
        n513 = Variant To Data(error in=w907, type=w909, Variant=w908) -> (data=w910:T39)  [unwired: 1 out]
        n514 = Unbundle By Name(w910) -> ()  [unwired: 1 out]
      }
      frame "Dwell Times" {
        n515 = Variant To Data(error in=w916, type=w914, Variant=w915) -> (data=w917:T39)  [unwired: 1 out]
        n516 = Unbundle By Name(w917) -> ("Procedure"=w913:T12)
        n517 = case shown="\"Test\"" w913 {
          tunnel: [w919 _] -> w912
          frame "Test" {
            w918 = u32 2 items=["Grayscale", "Binary", "Gradient", "Rainbow", "Temperature", "User Defined", "Binary 16 Bit", "Gradient 16 Bit", "Rainbow 16 Bit", "Temperature 16 Bit", "User Defined 16 Bit"] ("Palette:Palette Type")
            n518 = local read "Signal Channel"() -> (w922:enum16{"Red", "Green"})
            n519 = call "Test_Dwelltime.vi"("number of points"=4, "Signal Channel"=w922) -> ("error out"=w919:errorcluster, "MaxProj"=w921:T5)  [unwired: 8 in]
            n520 = property on="Image" class="ImageControl"(error in=w919, "Palette Type"=w918) -> ()  [unwired: 1 in, 2 out]
            n521 = local write "Image"(w921) -> ()
          }
          frame Default {
          }
        }
        n522 = call "Message_Update_Calib_frontpanel.vi"("error in (no error)"=w912, "Message"="Tested: Image is Updated") -> ()  [unwired: 9 in, 1 out]
      }
      frame "Magnification" {
        n523 = Variant To Data(type=w923, Variant=w925) -> (data=w924:T39)  [unwired: 1 in, 1 out]
        n524 = Unbundle By Name(w924) -> ()  [unwired: 1 out]
      }
    }
  }
  n525 = while {
    tunnel: w18 -> [w941]
    tunnel: w17 -> [w938]
    tunnel: [w936] -> w38
    tunnel: w22 -> [w931]
    tunnel: w13 -> [w929]
    stop <- w939 stop-if-true
    n526 = Dequeue Element(queue=w941, timeout in ms (-1)=250, error in (no error)=w938) -> (element=w940:T50, error out=w936:errorcluster)  [unwired: 2 out]
    n527 = case shown="\"Green\"" "Signal Channel" {
      tunnel: w940 -> [w943 w945]
      tunnel: [w942 w944] -> w928
      frame "Red", Default {
        n528 = Unbundle By Name(w943) -> ("Red channel"=w942:T5)
      }
      frame "Green" {
        n529 = Unbundle By Name(w945) -> ("Green channel"=w944:T5)
      }
    }
    n530 = local read "Visible(Grid)"() -> (w926:bool)
    n531 = local read "Grid Lines"() -> (w932:u32)
    n532 = Equal?(x=w928, y=T5 refnum) -> (x = y?=w933:bool)
    n533 = local read "Stop_Ind"() -> (w939:bool)
    n534 = case shown="False" w933 {
      tunnel: w928 -> [w949 w954]
      tunnel: w932 -> [w948 _]
      tunnel: [w947 w954] -> w927
      tunnel: w926 -> [w946 _]
      frame False {
        n535 = case shown="True" w946 {
          tunnel: w949 -> [w950 w953]
          tunnel: w948 -> [_ w952]
          tunnel: [w950 w951] -> w947
          frame False {
          }
          frame True {
            n536 = call "Draw_Grid.vi"("Grid Lines"=w952, "Image In"=w953) -> ("Image Out"=w951:T5)  [unwired: 8 in, 1 out]
          }
        }
      }
      frame True {
      }
    }
    "Image" <- w927
    n537 = call "IMAQ Copy"("error in (no error)"=w931, "Image Dst"=w929, "Image Src"=w928) -> ("error out"=→"error out 2":errorcluster)  [unwired: 3 in, 1 out]
  }
  n538 = while {
    tunnel: w21 -> [w985]
    tunnel: w20 -> [_]
    tunnel: w14 -> [w977]
    tunnel: w11 -> [w984]
    tunnel: w9 -> [w981]
    tunnel: w7 -> [_]
    tunnel: w5 -> [w961]
    stop <- w989 stop-if-true
    w978 = T53 0 items=["Use Bit Depth", "Shift", "Use Lookup Table"] ("Method")
    w980 = T18 0 items=["Grayscale (U8)", "Grayscale (I16)", "Grayscale (SGL)", "Complex (CSG)", "RGB (U32)", "HSL (U32)", "RGB (U64)", "Grayscale (U16)"] ("Image Type")
    n539 = call "IMAQ GetImageSize"("Image"=w977) -> ("Y Resolution"=→"Y Res.":i32, "X Resolution"=→"X Res.":i32)  [unwired: 3 in, 1 out]
    n540 = call "IMAQ ImageToArray"("Image"=w977) -> ("error out"=w983:errorcluster, "Image Pixels (I16)"=w968:i16[][])  [unwired: 3 in, 3 out]
    "error out 3" <- w983
    n541 = call "extract core.vi"("Y offset"="Y offset", "X offset"="X offset", "Core extraction size"="Core extraction size", "I/P array"=w968) -> ("O/P array"=w971:i16[][])  [unwired: 7 in]
    n542 = Transpose 2D Array(2D array=w968) -> (transposed array=w969:i16[][])
    n543 = for {
      tunnel: w969 -> [w1048] mode=indexing
      tunnel: [w1047] -> w967 mode=indexing
      n544 = Reverse 1D Array(array=w1048) -> (reversed array=w1047:i16[])
    }
    "Intensity" <- w967
    n545 = call "IMAQ ArrayToImage"("error in (no error)"=w983, "Image Pixels (I16)"=w971, "Image"=w985) -> ("error out"=w982:errorcluster, "Image Out"=w959:T5)  [unwired: 7 in]
    n546 = disable-structure shown="Disabled" {
      disable-tunnel: w961 -> [w1024 _]
      disable-tunnel: w959 -> [w1003 _]
      frame Disabled {
        w1002 = T18 0 items=["Grayscale (U8)", "Grayscale (I16)", "Grayscale (SGL)", "Complex (CSG)", "RGB (U32)", "HSL (U32)", "RGB (U64)", "Grayscale (U16)"] ("Image Type")
        n547 = call "IMAQ Copy"("Image Dst"=w1024, "Image Src"=w1003) -> ("error out"=w1001:errorcluster, "Image Dst Out"=w1000:T5)  [unwired: 4 in]
        n548 = Unbundle By Name("Core image filtered") -> ("Numeric"=w1009:dbl, "Numeric"=w1008:dbl)
        n549 = Bundle By Name(cluster=cluster{"Lower value":sgl, "Upper value":sgl} {"Lower value"=0.0, "Upper value"=0.0} ("Range (Threshold 1)"), "Lower value"=w1009, "Upper value"=w1008) -> (w1007:cluster{"Lower value":sgl, "Upper value":sgl})
        n550 = call <vilib>:"IVA Adjust Dynamic.vi"("Image Type"=w1002, "error in (no error)"=w1001, "Image Src"=w1000) -> ("error out"=w998:errorcluster, "Image Out"=w999:T5)  [unwired: 7 out]
        n551 = call "IMAQ Threshold"("error in (no error)"=w998, "Range"=w1007, "Image Src"=w999) -> ("error out"=w1005:errorcluster, "Image Dst Out"=w1006:T5)  [unwired: 3 in, 4 out]
        n552 = call "IMAQ Morphology"("Structuring Element"=i32[][] [[0, 1, 0], [1, 1, 1], [0, 1, 0]] ("Structuring Element (Basic Morphology 1) 2"), "Square/Hexa (Square)"=FALSE, "error in (no error)"=w1005, "Operation"="Operation", "Image Src"=w1006) -> ("error out"=w1020:errorcluster, "Image Dst Out"=w1019:T5)  [unwired: 5 in]
        n553 = call "IMAQ Find Circles"("Max Radius"=sgl 500.0, "error in (no error)"=w1020, "Min Radius"=sgl 3.0, "Image Src"=w1019) -> ("error out"=→"error out 6":errorcluster, "Circles Data"=w1018:T13, "Nb Circles"=w1012:i32, "Image Dst Out"=w1017:T5)  [unwired: 1 in, 3 out]
        "Nb Circles" <- w1012
        "Circles Data" <- w1018
        n554 = Greater Than 0?(x=w1012) -> (x > 0?=w1011:bool)
        n555 = case shown="True" w1011 {
          tunnel: w1018 -> [_ w1028]
          tunnel: w1017 -> [w1025 w1027]
          tunnel: [w1025 w1026] -> w1016
          frame False {
          }
          frame True {
            n556 = for {
              tunnel: w1028 -> [w1039] mode=indexing
              tunnel: w1027 -> [w1034]
              tunnel: [w1030] -> w1026
              n557 = Unbundle By Name(w1039) -> ("Pos. X"=w1038:i32, "Pos. Y"=w1037:i32, "Radius"=w1036:i32)
              n558 = Bundle By Name(cluster=T51 {"Center X"=0, "Center Y"=0, "Inner Radius"=0, "Outer Radius"=0, "Start Angle"=0.0, "End Angle"=0.0} ("Annulus"), "Center X"=w1038, "Center Y"=w1037, "Outer Radius"=w1036) -> (w1035:T51)
              n559 = call "IMAQ Convert Annulus to ROI"("Annulus"=w1035) -> ("ROI Descriptor"=w1033:T54)  [unwired: 8 in, 1 out]
              n560 = call "IMAQ Overlay ROI"("Colors (Green)"=u32[] [65280], "Group"="Circles", "Point Symbol"=u32[][] [[16777216, 16777216, 16777216, 16771584, 16777216, 16777216, 16777216], [16777216, 16777216, 16777216, 16771584, 16777216, 16777216, 16777216], [16777216, 16777216, 16777216, 16771584, 16777216, 16777216, 16777216], [16771584, 16771584, 16771584, 16771584, 16771584, 16771584, 16771584], [16777216, 16777216, 16777216, 16771584, 16777216, 16777216, 16777216], [16777216, 16777216, 16777216, 16771584, 16777216, 16777216, 16777216], [16777216, 16777216, 16777216, 16771584, 16777216, 16777216, 16777216]], "ROI Descriptor"=w1033, "Image"=w1034) -> ("Image Out"=w1030:T5)  [unwired: 5 in, 1 out]
            }
          }
        }
      }
      frame Enabled {
      }
    }
    n561 = Transpose 2D Array(2D array=w971) -> (transposed array=w972:i16[][])
    n562 = for {
      tunnel: w972 -> [w1050] mode=indexing
      tunnel: [w1049] -> w970 mode=indexing
      n563 = Reverse 1D Array(array=w1050) -> (reversed array=w1049:i16[])
    }
    "Core Intensity" <- w970
    n564 = call "IMAQ Copy"("Image Dst"=w981, "Image Src"=w959) -> ("Image Dst Out"=w979:T5)  [unwired: 4 in, 1 out]
    n565 = call "IMAQ Cast Image 2"("Image Src"=w979, "Method"=w978, "Image Dst"=w979, "Image Type"=w980) -> ("Image Dst Out"=w960:T5)  [unwired: 10 in, 1 out]
    n566 = case shown="\"Prewitt\"" "Filter Type" {
      tunnel: w960 -> [w1055 w1061 w1067 w1073 w1079 w1085 w1091]
      tunnel: w982 -> [w1054 w1060 w1066 w1072 w1078 w1084 w1090]
      tunnel: w984 -> [w1053 w1062 w1068 w1074 w1080 w1086 w1092]
      tunnel: [w1052 w1057 w1063 w1069 w1075 w1081 w1087] -> w987
      tunnel: [w1051 w1058 w1064 w1070 w1076 w1082 w1088] -> w958
      frame "Convolution", Default {
        n567 = call "IMAQ Convolute"("Kernel"=sgl[][] [[0.0, -1.0, 0.0], [-1.0, 0.0, 1.0], [0.0, 1.0, 0.0]], "error in (no error)"=w1054, "Image Dst"=w1053, "Image Src"=w1055) -> ("error out"=w1052:errorcluster, "Image Dst Out"=w1051:T5)  [unwired: 6 in]
      }
      frame "Differentiation" {
        n568 = call "IMAQ EdgeDetection"("Method"=T52."Differentiation", "error in (no error)"=w1060, "Image Dst"=w1062, "Image Src"=w1061) -> ("error out"=w1057:errorcluster, "Image Dst Out"=w1058:T5)  [unwired: 6 in]
      }
      frame "Gradient" {
        n569 = call "IMAQ EdgeDetection"("Method"=T52."Gradient", "error in (no error)"=w1066, "Image Dst"=w1068, "Image Src"=w1067) -> ("error out"=w1063:errorcluster, "Image Dst Out"=w1064:T5)  [unwired: 6 in]
      }
      frame "Prewitt" {
        n570 = call "IMAQ EdgeDetection"("Method"=T52."Prewitt", "error in (no error)"=w1072, "Image Dst"=w1074, "Image Src"=w1073) -> ("error out"=w1069:errorcluster, "Image Dst Out"=w1070:T5)  [unwired: 6 in]
      }
      frame "Roberts" {
        n571 = call "IMAQ EdgeDetection"("Method"=T52."Roberts", "error in (no error)"=w1078, "Image Dst"=w1080, "Image Src"=w1079) -> ("error out"=w1075:errorcluster, "Image Dst Out"=w1076:T5)  [unwired: 6 in]
      }
      frame "Sigma" {
        n572 = call "IMAQ EdgeDetection"("Method"=T52."Sigma", "error in (no error)"=w1084, "Image Dst"=w1086, "Image Src"=w1085) -> ("error out"=w1081:errorcluster, "Image Dst Out"=w1082:T5)  [unwired: 6 in]
      }
      frame "Sobel" {
        n573 = call "IMAQ EdgeDetection"("Method"=T52."Sobel", "error in (no error)"=w1090, "Image Dst"=w1092, "Image Src"=w1091) -> ("error out"=w1087:errorcluster, "Image Dst Out"=w1088:T5)  [unwired: 6 in]
      }
    }
    "Core Image Filtered" <- w958
    n574 = disable-structure shown="Enabled" {
      disable-tunnel: [w992 w997] -> w956
      disable-tunnel: w959 -> [w991 w997]
      disable-tunnel: "CH2" -> [w990 _]
      frame Enabled {
        n575 = case shown="True" w990 {
          tunnel: w991 -> [w993 w995]
          tunnel: [w993 w994] -> w992
          frame False {
          }
          frame True {
            n576 = call "Draw_Grid.vi"("Grid Lines"=u32 2, "Image In"=w995) -> ("Image Out"=w994:T5)  [unwired: 8 in, 1 out]
          }
        }
      }
      frame Disabled {
      }
    }
    "Core Image" <- w956
    n577 = call "IMAQ Histograph"("Image"=w956) -> ("Histogram Graph"=→"Histogram":T7)  [unwired: 7 in, 3 out]
    n578 = call "IMAQ Histograph"("error in (no error)"=w987, "Image"=w958) -> ("error out"=w963:errorcluster, "Mean Value"=w965:sgl)  [unwired: 6 in, 2 out]
    n579 = case shown="True" "Mov. Avg" {
      tunnel: w965 -> [w1042 w1046]
      tunnel: [w1042 w1045] -> w964
      tunnel: w963 -> [w1041 w1044]
      tunnel: [w1041 w1043] -> w962
      frame False {
      }
      frame True {
        n580 = call "Filter"("error in (no error)"=w1044, "Signal"=w1046) -> ("error out"=w1043:errorcluster, "Filtered Signal"=w1045:dynamicdata)  [unwired: 8 in]
      }
    }
    "Mean Value" <- w964
    "error out 4" <- w962
    n581 = local read "Stop_Ind"() -> (w989:bool)
    "New Image" <- w977
  }
  n582 = flat-sequence {
    tunnel: w26 -> [_]
    frame #0 {
      # "Enables live imaging windows again after the loop has stopped as the user has exited"
      n583 = global read "gl_UI Ctrl Refs.vi" "UI ctrl refs"() -> (w1095:T35)
      n584 = Unbundle By Name(w1095) -> ("Live Imaging"=w1094:refnum<vi>)
      n585 = property class="Bool (strict)"(reference=w1094, "DisabledEnum"=T22."Enabled" ("Disabled")) -> ()  [unwired: 1 in, 2 out]
    }
  }
  n586 = call <vilib>:"Clear Errors.vi"("error in (no error)"=w38) -> ()  [unwired: 5 in, 2 out]
  n587 = flat-sequence {
    tunnel: w40 -> [w1098]
    tunnel: w43 -> [w1099]
    tunnel: [w1099] -> w3
    tunnel: [w1098] -> w2
    tunnel: w1 -> [w1096]
    tunnel: w3 -> [w1101]
    tunnel: w2 -> [w1100]
    frame #0 {
      n588 = control-ref of="Objectives"() -> (w1097:refnum<vi>)
      n589 = call "Tree - Close reference.vi"("error in (no error)"=w1096, "TreeControl in"=w1097) -> ()  [unwired: 9 in, 1 out]
    }
    frame #1 {
      n590 = global write "General Globals.vi" "Calibration Toolbox"(w1100) -> ()
      "Stop_Ind" <- w1101
    }
    frame #2 {
      n591 = control-ref of="This VI"() -> (w1104:refnum<vi>)
      n592 = invoke class="VI" method="FP.Close"(reference=w1104, error in=errorcluster {"status"=FALSE, "code"=0, "source"=""} ("error in (no error)")) -> (error out=→"error out 9":errorcluster)  [unwired: 1 in, 2 out]
    }
  }
